vi "UHR-Fleezers Control (fpga) - avogadro 7 rm bd2.vi"() -> ()   [LabVIEW 2014]
doc: "UHR-Fleezers Instrument Control Code (fpga)"
uses:
  <vilib>/Platform/TimedLoop/XDataNode/timing_clust.ctl
  <vilib>/Platform/TimedLoop/XDataNode/nitl_modes.ctl
  <vilib>/Platform/TimedLoop/XDataNode/wakeup.ctl
  <vilib>/rvi/Emulation/niFpgaGetClockAttributes.vi
  <vilib>/rvi/Emulation/niFpgaSctlEmulationGetInTimedLoop.vi
  <vilib>/rvi/Emulation/niFpgaEmulationReportErrorSimple.vi
  <vilib>/rvi/Emulation/niFpgaProcessEmulError.vi
  <vilib>/rvi/eio/common/nirviEmuTemplateMethod_errors.vi
  <vilib>/rvi/interface/RandomDataEmulation/niFpgaRandomDataHandleErrors.vi
  <vilib>/rvi/Emulation/niFpgaCriticalErrorInLSC.vi
  <vilib>/rvi/Emulation/niFpgaEmulationIsFPGAContextNoSignature.vi
  <vilib>/rvi/errors/niFpgaSetErrorForExecOnDevCompSimple.vi
  <vilib>/rvi/eio/common/nirviEmuReportErrorAndStop.vi
  <vilib>/rvi/DataTransferAndStorage/Container/Common/niFpgaContainerGetUniqueNameForEmu.vi
  <vilib>/rvi/FIFO/Fifo_Resource/nirvififoEmulationSetSize.vi
  <vilib>/rvi/FIFO/Fifo_Resource/nirviFifoEmulationQueueMgr.vi
  <instcachedir>/0/nirviFifoEmulationQueueMgr_E5CAEC123FF24DC58D834DCA3CDAA9B5.lvgen/nirviFifoEmulationQueueMgr_E5CAEC123FF24DC58D834DCA3CDAA9B5_001.vi
  <vilib>/rvi/FIFO/Fifo_Resource/nirvififoEmulationDetermineInputValidOut.vi
  <vilib>/rvi/FIFO/Fifo_Resource/nirvififoEmulationCreateLock.vi
  <vilib>/rvi/FIFO/Fifo_Resource/nirvififoEmulationObtainLock.vi
  <vilib>/rvi/FIFO/Fifo_Resource/nirvififoEmulationReleaseLock.vi
  <vilib>/rvi/occurrence/nirviWaitOnOccurrenceBase.vi
  <vilib>/rvi/errors/nirviReportUnexpectedCaseInternalError.vi
  <vilib>/rvi/errors/nirviReportUnexpectedCaseInternalError (U32).vi
  <vilib>/rvi/DataTransferAndStorage/Container/Common/niFpgaContainerExecOnDevCompGetState.vi
  <vilib>/Utility/error.llb/Clear Errors.vi
  <vilib>/eio/EIONode/EIONode.xnode
  <vilib>/eio/EIOMethodNode/EIOMethodNode.xnode
  <vilib>/rvi/DataTransferAndStorage/Container/XNode/niFpgaContainer.xnode
  <vilib>/rvi/interface/RandomDataEmulation/nirviRandomDataFpgaReadWriteTemplate.vi
  <vilib>/rvi/FIFO/Fifo_Resource/nirvififoEmulationWrite.vi
  <vilib>/rvi/FIFO/Fifo_Resource/niFpgaFifoEmulationRefIn.vi
  <vilib>/addons/control/pid/fpga.llb/XNode/niFpgaPID.xnode
  <vilib>/Platform/TimedLoop/XDataNode/XDataNode.xnode
  <vilib>/rvi/FIFO/Fifo_Resource/nirvififoEmulationRead.vi
  <vilib>/Platform/TimedLoop/XDataNode/XDNodeRunTimeDep.lvlib
  <vilib>/rvi/Memory/Memory_Emulation/niFpgaMemoryEmulationRefIn.vi
panel:
  in  "BD 1 Delay (ticks)":u8
  out "lifetime (ticks)":u16
  in  "Lifetime to FIFO":bool
  in  "Tab Control":T1(tab)=enum."MCL trap control"
  in  "Set 3":bool
  in  "Set 2":bool=TRUE
  in  "Set 1":bool=TRUE
  in  "Trap Pos to FIFO":bool
  in  "N of AI1 Int Acq Sets":i16=2 min=1 max=3 step=1
  out "AI Late Counter":u8
  in  "ai count":u16=400
  in  "+ phase":bool
  in  "Phase count adjustment":i16
  out "Relative phase":i16
  in  "AI to FIFO":bool
  out "BD1 Frequency Out 1":u64
  out "BD1 Frequency Out 2":u64
  out "Trap Pos FIFO Timeout":u16
  out "Trap AI FIFO Timeout":u16
  in  "Trap FIFO Set Timeout":i32
  in  "Tab Control 2":T2(tab)
  in  "Multiple trap 3 position offset \nfile":bool
  in  "Piezo offset Y points":u64
  in  "Piezo offset X points":u64
  in  "Piezo offset Xmin":u64
  in  "Piezo Offset Ymin":u64
  in  "Piezo Offset Increment":u64
  out "BD1 amplitude 1 out":u16
  out "BD1 amplitude 2 out":u16
  in  "FB output range":cluster{"output low":i16, "output high":i16}={"output low"=0, "output high"=3000}
  in  "FB Gains":T3={"proportional gain (Kc)"=10, "integral gain (Kc*Ts/Ti)"=5, "derivative gain (Kc*Td/Ts)"=0}
  in  "RF synth green feedback max":i16=4000
  in  "RD":bool=TRUE
  in  "Swap F1 and F2":bool
  in  "Cont. Scan":bool
  in  "Abort scan":bool
  in  "Cycles per step":u64
  in  "Scan BD":bool
  in  "Number of scans":u16
  in  "Scan steps":u64
  in  "Scan freq.  increment":i64
  out "Scanning":bool
  in  "Start scan":bool
  in  "OSK Bd 1":bool
  in  "Reset Bd 1":bool
  in  "PMODE":bool=TRUE
  in  "Number Interlace Cycles":u8=2 min=1 max=3
  in  "Interlace Off Parameters":u8=1 min=1 max=3
  in  "Interlace ON/OFF":bool
  out "DIO Relative phase":i16
  in  "Phase count adjustment (DIO)":i16
  in  "+ phase (DIO)":bool
  out "DIO Late Counter":u8
  in  "DIO count 1 (ticks)":u16=400
  in  "DIO count 2 (ticks)":u16=400
  in  "DIO count 3 (ticks)":u16=400
  out "AI2 Y Sum Set 2":i16
  out "AI2 Y Sum Set 1":i16
  in  "FB Setpoint Set 1":i16 min=0 step=1
  in  "FB Reset Set 1":bool
  in  "FB On/Off Set 1":bool
  in  "FB Reset Set 2":bool
  in  "FB On/Off Set 2":bool
  in  "FB Setpoint Set 2":i16 min=0 step=1
  out "Scan I":u64
  in  "Amp switch delay":u8=5
  in  "RF synth bd controls green":bool
  in  "Phase Trap 2":fxp<+,14,14>
  in  "Phase Trap 1":fxp<+,14,14>
  in  "Phase offset method":u8
  in  "BD 1 Amplitude 1":u16
  in  "BD 1 Frequency 1":u64
  in  "BD 1 Amplitude 2":u16
  in  "BD 1 Frequency 2":u64
  in  "BD 1 Amplitude 3":u16
  in  "BD 1 Frequency 3":u64
  in  "Next trap write delay (ticks)":u8 caption="Count(Ticks)"
  out "Random phase generated":fxp<+,14,14>
  in  "RF phase reset before cycles":bool
  in  "Ready Write":bool
  in  "Data":i64
  in  "Address 2":u32
  out "Piezo X out":i16
  out "Piezo Y out":i16
  in  "Piezo Trap ON/Off (AO3)":i16
  in  "Piezo Trap X (AO5)":i16
  in  "Piezo Trap Y (AO4)":i16
  in  "Symmetric force feedback\nand raster scan":bool
  in  "FB Min frequency":u64
  in  "FB Max Frequency":u64
  in  "Dynamic Force FB (Ronen)":bool
  in  "Trap pos. FB Range":T4={"FB2 output low"=-1.0, "FB2 output high"=0.999969482421875}
  in  "Trap Pos. FB Gains":T5={"proportional gain (Kc)"=0.999969482421875, "integral gain (Kc*Ts/Ti)"=0.999969482421875, "derivative gain (Kc*Td/Ts)"=0.0}
  in  "B factor":fxp<+/-,32,16>
  in  "Negate Diff?":bool
  in  "Diff FB Measurement?":bool
  in  "FB Trig Integrate":u32=1
  out "TTrig?":bool
  in  "TTrig Negate Pos":bool=TRUE
  out "Trap Pos FB Int Signal":fxp<+/-,24,9> format="%.18g"
  out "Trap Pos FB Int-Norm Signal":fxp<+/-,16,1> format="%.16g"
  in  "FPGA TTrig Thresh":i64
  in  "FPGA Trap Trig":bool
  out "Trap Pos FB Action":i64
  in  "Trap Pos. FB Offset Factor":i64
  in  "Trap Pos. FB Mult Factor":i64=2
  in  "Trap Pos. FB Reset":bool
  in  "Trap Pos FB Monitor T1 or T2":bool
  in  "AI1 X Scale":u16
  in  "Trap Pos FB Int Count":u16=100
  in  "Trap Pos FB Negate Action":bool
  out "AI1 X Set 2":fxp<+/-,16,1>
  out "AI1 X Set 1":fxp<+/-,16,1>
  in  "Trap Pos. FB SP":fxp<+/-,16,1>
  in  "Force feedback":bool
  out "TTrig Sig":i64
  out "TTrig Fin Thresh":i64
  in  "ScanTrap 3 or Fl-laser":bool
  in  "1D or 2D Scan?":bool
  in  "Abort scan (MCL)":bool
  in  "MCL Scan Axis":bool
  in  "Cont. Scan (MCL)":bool
  out "Scan I (MCL)":u64
  in  "Number of scans (MCL)":u16
  out "Scanning MCL":bool
  in  "Scan steps (MCL)":u64
  in  "Cycles per step (MCL)":u64
  in  "Scan freq.  increment (MCL)":i16
  in  "Start scan (MCL)":bool
  in  "AO2 (X)":i16
  in  "AO1 (Y)":i16
  out "MCL Late Counter":u8
  in  "MCL count":u32=800
  out "MCL Relative Phase":i16
  in  "Phase count adjustment (MCL)":i16
  in  "+ phase (MCL)":bool
  in  "Lifetime events to read blue":u16=100
  in  "Lifetime read blue fifo":bool
  out "lifetime events in fifo":u16
  out "APD2 int gate":bool
  out "APD3 out state":bool
  in  "APD Gate Operating Mode":u8 max=2 step=1
  in  "Invert APD Gate":bool
  in  "APD Gate OFF Count":u16=100
  in  "APD Gate ON Count":u16=300
  out "APD 1 Gate Late Counter":u8
  out "APD 1 Gate Relative Phase":i16
  in  "Phase count adjustment (APD 1 Gate)":i16
  in  "+ phase (APD 1 Gate)":bool
  out "APD 2 Counts 0":u32
  out "APD 2 Counts 1":u32
  out "APD 1 Counts 0":u32
  out "APD 1 Counts 1":u32
  out "APD1 out state":bool
  in  "APD AO scale factor":i16=1
  in  "APD to FIFO":bool
  in  "APD Acq Rate Count":u32=20000000
  out "APD Acq Late Counter":u8
  out "APD Acq Relative Phase":i16
  in  "Phase Count Adjustment (APD Acq)":i16
  in  "+ phase (APD Acq)":bool
  in  "Phase count adjustment (APD 2 Gate)":i16
  out "APD 2 Gate Late Counter":u8
  out "APD 2 Gate Relative Phase":i16
  in  "+ phase (APD 2 Gate)":bool
  out "APD2 out state":bool
  out "APD 3 Counts 0":u32
  out "APD 3 Counts 1":u32
  out "APD 3 Gate Late Counter":u8
  in  "Phase count adjustment (APD 3 Gate)":i16
  out "APD 3 Gate Relative Phase":i16
  in  "+ phase (APD 3 Gate)":bool
  out "APD1 int gate":bool
  out "APD3 int gate":bool
  in  "Lifetime timeout APD1":u16=200
  in  "Laser choice 2":u8=100
  in  "Laser choice 1":u8=100
  in  "Laser choice 0":u8=100
  in  "FL interlace OFF count 2":u16=100
  in  "FL interlace OFF count 1":u16=100
  in  "FL interlace ON count 2":u16=300
  in  "Fl interlace ON count 1":u16=300
  in  "D3 2":i16
  in  "I3 2":i16=5
  in  "P3 2":i16=10
  in  "Green FB Setpoint 2":i16=250 min=0 step=1
  in  "Green FB Reset 2":bool
  in  "D3":i16
  in  "I3":i16=5
  in  "P3":i16=10
  in  "Green Filter Flipper":bool
  in  "Green FB Count":u16=1200
  out "Green Late Counter":u8
  out "Green FB Relative Phase":i16
  in  "Phase count adjustment (Green FB)":i16=10
  in  "+ phase (Green FB)":bool
  out "Green FB Sum":i16
  in  "Green int current ON count adj":u16=150
  in  "Current Out":u16=30000
  in  "Green FB On/Off":bool
  in  "Green FB Setpoint":i16=250 min=0 step=1
  in  "Green FB Reset":bool
  in  "Operating Mode 2":u8=2 max=2 step=1
  in  "Invert GI 2":bool
  in  "Green interlace OFF count 2":u16=900
  in  "Green interlace ON count 2":u16=300
  out "GI Late Counter 2":u8
  out "GI Relative phase 2":i16
  in  "Phase count adjustment (GI) 2":i16=20
  in  "+ phase (GI) 2":bool
  in  "FL interlace OFF count 0":u16=100
  out "GI Relative phase":i16
  in  "Phase count adjustment (GI)":i16
  in  "+ phase (GI)":bool
  in  "FL interlace ON count 0":u16=300
  out "GI Late Counter":u8
  in  "Invert GI":bool
  in  "Operating Mode":u8 max=2 step=1
  out "green FB running":bool
  in  "+ phase (RI)":bool
  out "RI Relative phase":i16
  out "RI Late Counter":u8
  in  "Red interlace ON count":u16=300
  in  "Red interlace OFF count":u16=100
  in  "Invert RI":bool
  in  "Red Laser Operating Mode":u8 max=2 step=1
  in  "Phase count adjustment (RI)":i16
  out "Red FB Intensity":i16
  in  "RI Current Out":u16=30000
  in  "Red FB On/Off":bool
  in  "D4":i16
  in  "I4":i16=5
  in  "P4":i16=10
  in  "Red FB Setpoint":i16=250 min=0 step=1
  in  "Red FB Reset":bool
  in  "RI Operating Mode 2":u8=2 max=2 step=1
  in  "Invert RI 2":bool
  in  "Phase count adjustment (BI AO)":i16=20
  in  "Blue current ON count adj (AO)":u16=150
  in  "BI Current Out":i16=30000
  in  "Blue FB On/Off":bool
  in  "D5":i16
  in  "I5":i16=5
  in  "P5":i16=10
  in  "Blue FB Setpoint":i16=250 min=0 step=1
  in  "Blue FB Reset":bool
  in  "BI Operating Mode (AO)":u8=2 max=2 step=1
  in  "Invert BI (AO)":bool
  in  "Blue OFF count (AO)":u16=900
  in  "Blue ON count (AO)":u16=300
  out "BI Late Counter (AO)":u8
  out "BI Relative phase (AO)":i16
  in  "+ phase (BI AO)":bool
  in  "Phase count adjustment (BI D)":i16
  in  "Blue Laser Operating Mode (D)":u8 max=2 step=1
  in  "Invert BI (D)":bool
  in  "Blue interlace OFF count (D)":u16=100
  in  "Blue interlace ON count (D)":u16=300
  out "Blue Late Counter (D)":u8
  out "BI Relative phase (D)":i16
  in  "+ phase (BI D)":bool
  out "Blue Intensity":i16
  in  "Invert EMCCD Gate":bool
  in  "EMCCD Gate ON count":u16=300
  in  "EMCCD Gate OFF count":u16=100
  out "EMCCD Late counter":u8
  out "EMCCD relative phase":i16
  in  "+ phase (EMCCD Gate)":bool
  in  "EMCCD Gate Operating Mode":u8 max=2 step=1
  in  "Phase Count Adjustment EMCCD Gate":i16
  # "Raster Scan AOD"
  # "1 (X)"
  # "2 (Y)"
  # "IR Intensity Feedback (RF BD 1)"
  # "FB Gains Set 1"
  # "FB output range 1"
  # "IR Intensity Feedback (RF BD 2) -\nonly when using BD 2 for green laser AOM (not trap Y)"
  # "Keep below 4096 (12 bits) to stay within range of RF board. Going over doesn't saturate, it truncates higher bits."
  # "RF phase offset control"
  # "Methods are:\n0 - Default, do nothing at all (no phase offset writes)\n1 - Manual phase adjustment\n2 - Cycle the phase adjustment using the input phase numbers as increment values for each cycle"
  # "False is usual, True is external loop method"
  # "Parameters if using the external RF switching loop"
  # "Parameters if using the usual internal RF switching method"
  # "FB Triggering Excitation Laser"
  # "Trap Pos. FB Gains"
  # "Trap Pos. FB Range"
  # "AO1 (Y)"
  # "2D"
  # "Trap 3"
  # "1D"
  # "AO2 (X)"
  # "Fl Laser"
  # "APD AO for aligning"
  # "Detection Loop"
  # "Green fluorescent laser digital gate interlacing loop"
  # "0 Forced ON\n1 Forced OFF\n2 Interlacing"
  # "ALEX settings:"
  # "Controls for usual IA ME controls green AOM"
  # "Controls for RF synth board controls green AOM"
  # "Green FB Gains"
  # "Red fluorescent laser digital gate interlacing loop"
  # "Detection Loop"
  # "0 Forced ON\n1 Forced OFF\n2 Interlacing"
  # "Analog/FB Control Loop\n(Disabled)"
  # "Digital Control Loop"
  # "Blue laser intensity reading"
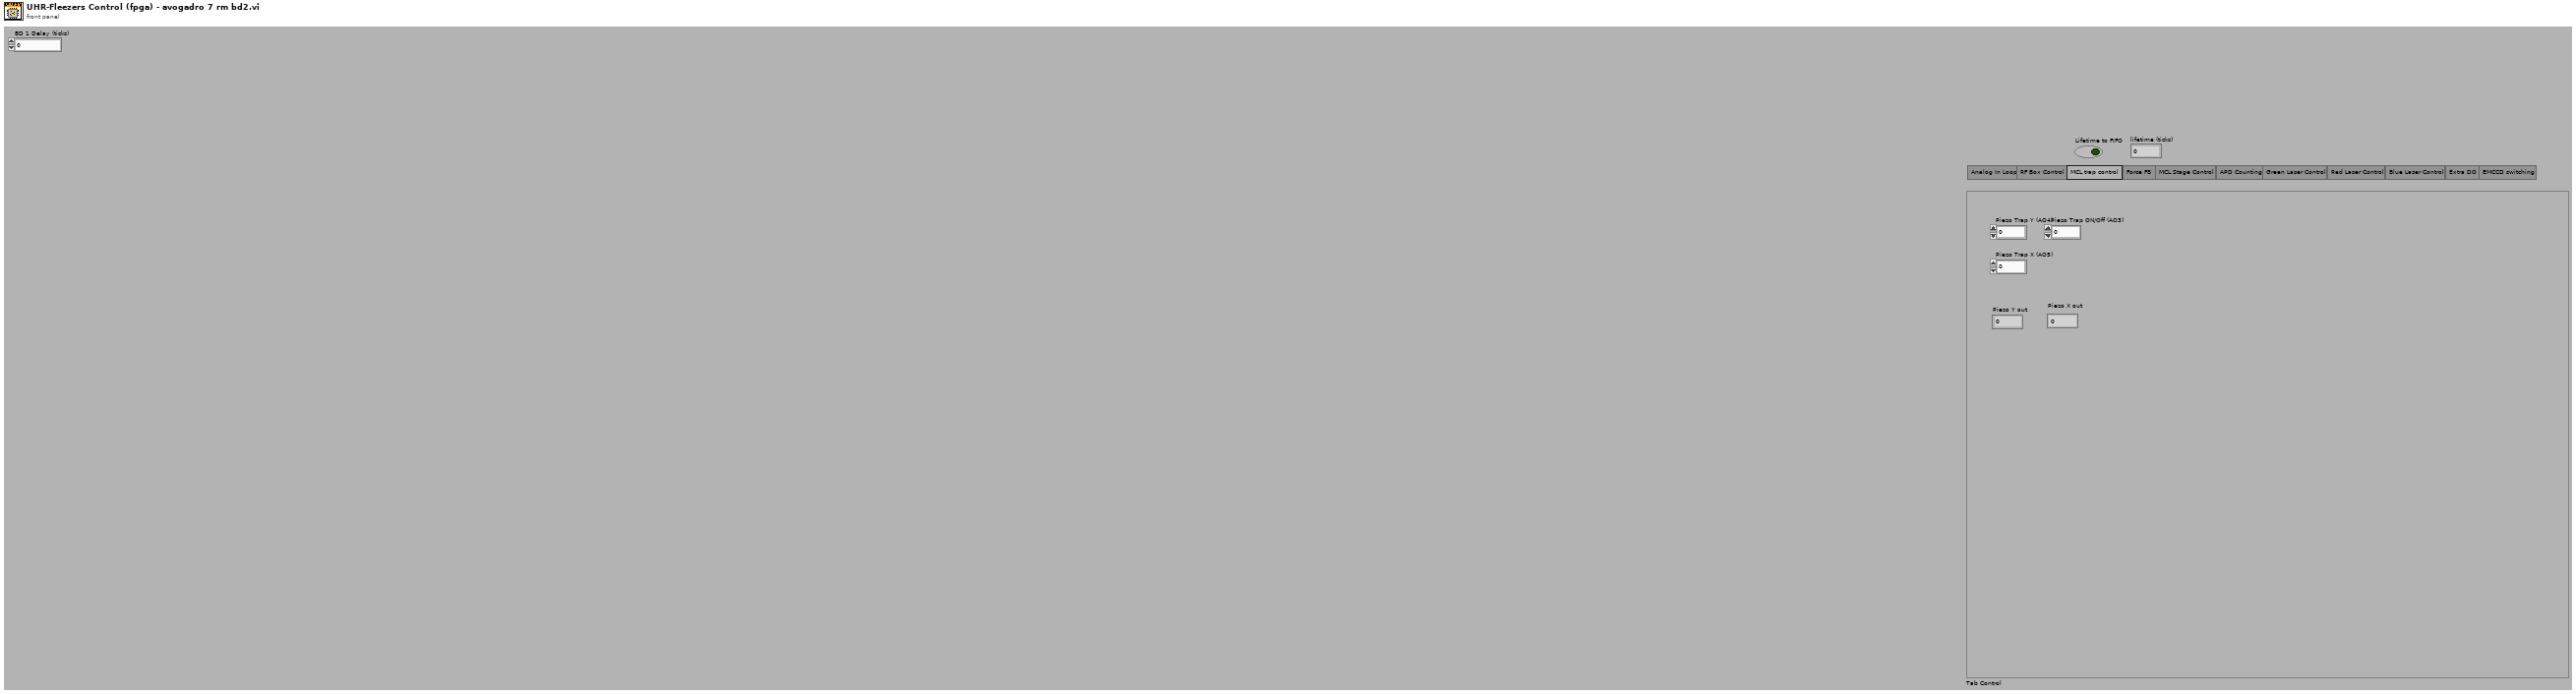
[diagram p1: front panel]
types:
  T1 = enum32{"Analog In Loop", "RF Box Control", "MCL trap control", "Force FB", "MCL Stage Control", "APD Counting", "Green Laser Control", "Red Laser Control", "Blue Laser Control", "Extra DO", "EMCCD switching"}
  T2 = enum32{"Controls", "Interlacing Frequency and Amplitude Values", "Oscillate trap from memory"}
  T3 = cluster{"proportional gain (Kc)":i16, "integral gain (Kc*Ts/Ti)":i16, "derivative gain (Kc*Td/Ts)":i16}
  T4 = cluster{"FB2 output low":fxp<+/-,16,1>, "FB2 output high":fxp<+/-,16,1>}
  T5 = cluster{"proportional gain (Kc)":fxp<+/-,16,1>, "integral gain (Kc*Ts/Ti)":fxp<+/-,16,1>, "derivative gain (Kc*Td/Ts)":fxp<+/-,16,1>}
  T6 = typedef "XDNodeRunTimeDep.lvlib/timing_clust.ctl" = cluster{"Expected End [f-1]":u64, "Actual End [f-1]":u64, "Finished Late? [f-1]":bool, "Expected End [i-1]":u64, "Actual End [i-1]":u64, "Finished Late? [i-1]":bool, "Expected Start [i]":u64, "Actual Start [i]":u64, "Expected Start [f]":u64, "Actual Start [f]":u64, "Source Name":string, "Structure Name":string, "Period":i64, "Deadline":i64, "Offset":i64, "Start":i64, "Priority":i32, "Timeout":i32, "Mode":T7, "Wakeup Reason":T8, "Error":errorcluster, "Source Type":string, "Secondary Source Type":string, "Global End Time":u64, "Global Start Time":u64, "Frame Duration":u64, "Iteration Duration":u64, "Assigned CPU":i32, "I/O Scan Engine Mode":u32}
  T7 = typedef "XDNodeRunTimeDep.lvlib/nitl_modes.ctl" = enum32{"No Change", "Process missed periods, maintain original phase", "Discard missed periods, maintain original phase", "Process missed periods, ignore original phase", "Discard missed periods, ignore original phase"}
  T8 = typedef "XDNodeRunTimeDep.lvlib/wakeup.ctl" = enum32{"Normal", "Aborted", "Asynchronous wakeup", "Timing source error", "Timed loop error", "Timeout"}
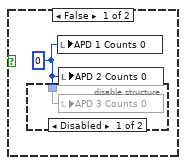
[diagram p4: hidden frame]
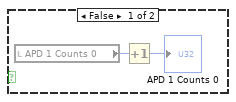
[diagram p9: hidden frame]
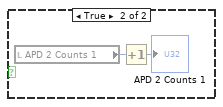
[diagram p11: hidden frame]
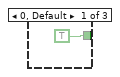
[diagram p13: hidden frame]
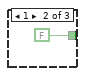
[diagram p14: hidden frame]
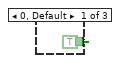
[diagram p15: hidden frame]
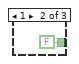
[diagram p16: hidden frame]
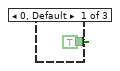
[diagram p18: hidden frame]
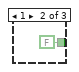
[diagram p19: hidden frame]
diagram:
  w11 = i16 0
  w15 = FALSE
  # "EMCCD gating"
  # "BD2 amp"
  # "BD1 amp"
  # "BD2 amp"
  # "BD1 amp"
  # "timing array current index"
  # "timing array"
  # "timing counter (phase adjusted here)"
  # "late counter"
  n1 = disable-structure shown="Disabled" {
    frame Disabled {
      w16 = i16 2 items=["UnSet Ready", "ReadWrite", "Wait Ready"]
      n2 = while "Handshake memory transfer for trap oscillation sin wave data" {
        shift-right: [w18] -> _
        shift-left: w16 -> [w19]
        stop <- FALSE stop-if-true
        # "Write"
        n3 = case shown="1" w19 {
          tunnel: [w22 w27 w28] -> w18
          frame 3, Default {
            w20 = i16 2 items=["UnSet Ready", "ReadWrite", "Wait Ready"]
            w21 = i16 1 items=["UnSet Ready", "ReadWrite", "Wait Ready"]
            n4 = Select(t=w21, s="Ready Write", f=w20) -> (s? t:f=w22:i16)
          }
          frame 1 {
            w27 = i16 0 items=["UnSet Ready", "ReadWrite", "Wait Ready"]
            n5 = xnode ("Memory Write")("Address"="Address 2", "Data"="Data", "Memory In"=refnum<k21> "Trap osc memory") -> ()  [unwired: 1 out]
          }
          frame 0 {
            w28 = i16 2 items=["UnSet Ready", "ReadWrite", "Wait Ready"]
            n6 = local write "Ready Write"(FALSE ("Ready Read")) -> ()
          }
        }
      }
    }
    frame Enabled {
    }
  }
  n7 = flat-sequence "FPGA initialization to do before running any of the loops" {
    tunnel: [u16 0 ("DIO count 3 (ticks)")] -> w4
    tunnel: [w34] -> _
    frame #0 {
      # "UDCLK out enable and set low"
      # "WR"
      # "BD 1"
      # "With the RF synth board initialization now done in a separate fpga vi, now when this vi is started, board is already configured and is ready for interlacing. Just need to set WR high and enabled UDCLK as write and set to low.\nbefore setting data and address bits."
      # "Start up expansion chassis early\nto avoid delays later"
      # "Set data and address values to something safe (a correct setting) so any initial WR and udclk flipping doesn't have a chance to mess anything up. Safe would be setting an unused data entry:"
      n8 = xnode "FPGA I/O Method Node"("Enable"=TRUE) -> ("FPGA I/O Out"=w31:refnum<k21>)  [unwired: 1 in]
      n9 = xnode "FPGA I/O Node"("Chassis2/Mod1/AO0"=u16 0 ("Chassis2/Mod4/AO0")) -> ("Chassis2/Mod2/AI0"=w34:i16)  [unwired: 2 in, 2 out]
      n10 = xnode "FPGA I/O Node"("Connector1/DIO15"=TRUE) -> ()  [unwired: 1 in, 1 out]
      n11 = xnode "FPGA I/O Node"("I/O Item"=FALSE ("Connector1/DIO30"), "FPGA I/O In"=w31) -> ()  [unwired: 1 out]
      n12 = xnode "FPGA I/O Node"("Connector1/DIO0"=FALSE, "Connector1/DIO1"=FALSE, "Connector1/DIO2"=FALSE, "Connector1/DIO3"=FALSE, "Connector1/DIO4"=FALSE, "Connector1/DIO5"=FALSE, "Connector1/DIO6"=FALSE, "Connector1/DIO7"=FALSE, "Connector1/DIO8"=FALSE, "Connector1/DIO9"=FALSE, "Connector1/DIO10"=FALSE, "Connector1/DIO11"=FALSE, "Connector1/DIO12"=FALSE, "Connector1/DIO13"=FALSE) -> ()  [unwired: 14 in, 14 out]
    }
  }
  n13 = node-c288() -> (w7:T6)  [unwired: 1 in]
  n14 = timed-loop "RF box board DIO control: control bits" {
    timing: w7 -> [_]
    timing-out: [_] -> w6
    tunnel: [w53] -> _
    tunnel: w4 -> [w53]
    stop <- FALSE stop-if-true
    n15 = xnode "FPGA I/O Node"("Connector1/DIO16"="RD", "Connector1/DIO17"="PMODE", "Connector1/DIO18"="OSK Bd 1", "Connector1/DIO19"="Reset Bd 1", "Connector0/DIO3"="Green Filter Flipper") -> ()  [unwired: 5 in, 5 out]
  }
  n16 = node-c288(w6) -> ()
  n17 = local read "AO1 (Y)"() -> (w13:i16)
  n18 = local read "AO2 (X)"() -> (w12:i16)
  n19 = To Unsigned Long Integer(number=w4) -> (unsigned 32bit integer=w3:u32)
  n20 = disable-structure shown="Disabled" {
    disable-tunnel: w4 -> [w61 _]
    disable-tunnel: [w60 _] -> w5
    frame Disabled {
      w60 = FALSE
      n21 = while "APD 1 Gating" {
        shift-right: [w116] -> _
        shift-left: w61 -> [w121]
        shift-right: [w115] -> _
        shift-left: w60 -> [w113]
        stop <- FALSE stop-if-true
        n22 = flat-sequence {
          tunnel: w121 -> [w124]
          tunnel: [w125] -> w119
          tunnel: [w124] -> w117
          tunnel: [w123] -> w114
          tunnel: w113 -> [w123]
          tunnel: [w128] -> w120
          tunnel: w119 -> [w128]
          tunnel: [w127] -> w118
          tunnel: w117 -> [w127]
          tunnel: w114 -> [w126]
          tunnel: [w146] -> w116
          tunnel: w120 -> [w160]
          tunnel: w118 -> [w157]
          tunnel: [w129] -> w115
          frame #0 {
            n23 = call "Loop Timer7"("Count(Ticks)"=w124) -> ("Tick Count(Ticks)"=w125:u16)
          }
          frame #1 {
            # "Signal maybe then sent through \na transistor before APD"
            n24 = xnode "FPGA I/O Node"("Connector0/DIO0"=w126) -> ()  [unwired: 1 in, 1 out]
            "APD1 int gate" <- w126
          }
          frame #2 {
            n25 = feedback #1(TRUE) -> (w152:bool)
            n26 = feedback-in #2(w160) -> ()
            n27 = feedback #2(w160) -> (w159:u16)
            n28 = Not(x=w152) -> (.not. x?=w149:bool)
            n29 = feedback-in #1(w149) -> ()
            n30 = Subtract(x=w160, y=w159) -> (x-y=w158:u16)
            n31 = Select(t="APD Gate ON Count", s=w149, f="APD Gate OFF Count") -> (s? t:f=w154:u16)
            n32 = Subtract(x=w158, y=w157) -> (x-y=w134:u16)
            n33 = Subtract(x=w154, y=w134) -> (x-y=w145:u16)
            n34 = Number To Boolean Array(number=w134) -> (Boolean array=w135:bool[])
            n35 = Or Array Elements(Boolean array=w135) -> (logical OR=w133:bool)
            n36 = Boolean To (0,1)(Boolean="+ phase (APD 1 Gate)") -> (0, 1=w143:i16)
            n37 = Boolean To (0,1)(Boolean=w133) -> (0, 1=w140:i16)
            n38 = Multiply(x=w143, y="Phase count adjustment (APD 1 Gate)") -> (x*y=w141:i16)
            n39 = To Unsigned Byte Integer(number=w140) -> (unsigned 8bit integer=w137:u8)
            n40 = Add(x=w145, y=w141) -> (x+y=w146:u16)
            n41 = feedback #3(i16 0) -> (w148:i16)
            n42 = Subtract(x=w148, y=w141) -> (x-y=w147:i16)
            "APD 1 Gate Relative Phase" <- w147
            n43 = feedback-in #3(w147) -> ()
            n44 = feedback #4(u8 0) -> (w138:u8)
            n45 = Add(x=w137, y=w138) -> (x+y=w136:u8)
            "APD 1 Gate Late Counter" <- w136
            n46 = feedback-in #4(w136) -> ()
            n47 = case shown="2" "APD Gate Operating Mode" {
              tunnel: [TRUE FALSE w163] -> w130
              tunnel: w152 -> [_ _ w163]
              frame 0, Default {
              }
              frame 1 {
              }
              frame 2 {
              }
            }
            n48 = Not(x=w130) -> (.not. x?=w131:bool)
            n49 = Select(t=w131, s="Invert APD Gate", f=w130) -> (s? t:f=w129:bool)
          }
        }
      }
      n50 = while "APD 2 Gating" {
        shift-right: [w65] -> _
        shift-left: w61 -> [w70]
        shift-right: [w64] -> _
        shift-left: w60 -> [w62]
        stop <- FALSE stop-if-true
        n51 = flat-sequence {
          tunnel: w70 -> [w73]
          tunnel: [w74] -> w68
          tunnel: [w73] -> w66
          tunnel: [w72] -> w63
          tunnel: w62 -> [w72]
          tunnel: [w77] -> w69
          tunnel: w68 -> [w77]
          tunnel: [w76] -> w67
          tunnel: w66 -> [w76]
          tunnel: w63 -> [w75]
          tunnel: [w99] -> w65
          tunnel: w69 -> [w109]
          tunnel: w67 -> [w107]
          tunnel: [w78] -> w64
          frame #0 {
            n52 = call "Loop Timer8"("Count(Ticks)"=w73) -> ("Tick Count(Ticks)"=w74:u16)
          }
          frame #1 {
            # "Signal maybe then sent through \na transistor before APD"
            n53 = xnode "FPGA I/O Node"("Connector0/DIO1"=w75) -> ()  [unwired: 1 in, 1 out]
            "APD2 int gate" <- w75
          }
          frame #2 {
            n54 = local read "APD Gate ON Count"() -> (w92:u16)
            n55 = local read "APD Gate OFF Count"() -> (w91:u16)
            n56 = feedback #5(TRUE) -> (w104:bool)
            n57 = feedback-in #6(w109) -> ()
            n58 = feedback #6(w109) -> (w93:u16)
            n59 = Not(x=w104) -> (.not. x?=w102:bool)
            n60 = feedback-in #5(w102) -> ()
            n61 = Subtract(x=w109, y=w93) -> (x-y=w108:u16)
            n62 = Select(t=w92, s=w102, f=w91) -> (s? t:f=w106:u16)
            n63 = Subtract(x=w108, y=w107) -> (x-y=w84:u16)
            n64 = Subtract(x=w106, y=w84) -> (x-y=w98:u16)
            n65 = Number To Boolean Array(number=w84) -> (Boolean array=w83:bool[])
            n66 = Or Array Elements(Boolean array=w83) -> (logical OR=w82:bool)
            n67 = Boolean To (0,1)(Boolean="+ phase (APD 2 Gate)") -> (0, 1=w96:i16)
            n68 = Multiply(x=w96, y="Phase count adjustment (APD 2 Gate)") -> (x*y=w94:i16)
            n69 = Boolean To (0,1)(Boolean=w82) -> (0, 1=w89:i16)
            n70 = Add(x=w98, y=w94) -> (x+y=w99:u16)
            n71 = To Unsigned Byte Integer(number=w89) -> (unsigned 8bit integer=w86:u8)
            n72 = feedback #7(i16 0) -> (w101:i16)
            n73 = Subtract(x=w101, y=w94) -> (x-y=w100:i16)
            "APD 2 Gate Relative Phase" <- w100
            n74 = feedback-in #7(w100) -> ()
            n75 = feedback #8(u8 0) -> (w87:u8)
            n76 = Add(x=w86, y=w87) -> (x+y=w85:u8)
            "APD 2 Gate Late Counter" <- w85
            n77 = feedback-in #8(w85) -> ()
            n78 = local read "APD Gate Operating Mode"() -> (w90:u8)
            n79 = case shown="2" w90 {
              tunnel: [TRUE FALSE w112] -> w79
              tunnel: w104 -> [_ _ w112]
              frame 0, Default {
              }
              frame 1 {
              }
              frame 2 {
              }
            }
            n80 = local read "Invert APD Gate"() -> (w81:bool)
            n81 = Not(x=w79) -> (.not. x?=w80:bool)
            n82 = Select(t=w80, s=w81, f=w79) -> (s? t:f=w78:bool)
          }
        }
      }
    }
    frame Enabled {
    }
  }
  n83 = disable-structure shown="Disabled" {
    disable-tunnel: w4 -> [w164 _]
    frame Disabled {
      n84 = while "Excitation laser intensity feedback measurement (all lasers)" {
        shift-right: [w165] -> _
        shift-left: w164 -> [w170]
        stop <- FALSE stop-if-true
        n85 = flat-sequence {
          tunnel: w170 -> [w172]
          tunnel: [w173] -> w168
          tunnel: [w172] -> w166
          tunnel: [w179] -> w169
          tunnel: w168 -> [w179]
          tunnel: [w178] -> w167
          tunnel: w166 -> [w178]
          tunnel: [w191] -> w165
          tunnel: w169 -> [w202]
          tunnel: w167 -> [w199]
          frame #0 {
            n86 = call "Loop Timer9"("Count(Ticks)"=w172) -> ("Tick Count(Ticks)"=w173:u16)
          }
          frame #1 {
            # "Design note:\n\nAll lasers need to be measured at the same \ntime because the AI expansion module\ncannot independently time the measurements\nwithin our requirements: there is dead time.\n\nThis probably wouldn't be an issue with the built\nin AI on the fpga board itself."
            n87 = xnode "FPGA I/O Node"("Connector1/DIO35"=TRUE) -> ("Chassis2/Mod1/AI2"=→"Blue Intensity", "Chassis2/Mod1/AI1"=→"Red FB Intensity", "Chassis2/Mod1/AI0"=→"Green FB Sum")  [unwired: 4 in, 4 out]
          }
          frame #2 {
            n88 = feedback-in #9(w202) -> ()
            n89 = feedback #9(w202) -> (w201:u16)
            n90 = Subtract(x=w202, y=w201) -> (x-y=w200:u16)
            n91 = xnode "FPGA I/O Node"("Connector1/DIO35"=FALSE) -> ()  [unwired: 1 in, 1 out]
            n92 = Subtract(x=w200, y=w199) -> (x-y=w181:u16)
            n93 = Subtract(x="Green FB Count", y=w181) -> (x-y=w195:u16)
            n94 = Number To Boolean Array(number=w181) -> (Boolean array=w182:bool[])
            n95 = Or Array Elements(Boolean array=w182) -> (logical OR=w180:bool)
            n96 = Boolean To (0,1)(Boolean="+ phase (Green FB)") -> (0, 1=w193:i16)
            n97 = Boolean To (0,1)(Boolean=w180) -> (0, 1=w187:i16)
            n98 = Multiply(x=w193, y="Phase count adjustment (Green FB)") -> (x*y=w188:i16)
            n99 = Add(x=w195, y=w188) -> (x+y=w191:u16)
            n100 = To Unsigned Byte Integer(number=w187) -> (unsigned 8bit integer=w184:u8)
            n101 = feedback #10(i16 0) -> (w190:i16)
            n102 = Subtract(x=w190, y=w188) -> (x-y=w189:i16)
            "Green FB Relative Phase" <- w189
            n103 = feedback-in #10(w189) -> ()
            n104 = feedback #11(u8 0) -> (w185:u8)
            n105 = Add(x=w184, y=w185) -> (x+y=w183:u8)
            "Green Late Counter" <- w183
            n106 = feedback-in #11(w183) -> ()
          }
        }
      }
    }
    frame Enabled {
    }
  }
  n107 = disable-structure shown="Disabled" {
    disable-tunnel: w4 -> [w203 _]
    frame Disabled {
      n108 = while "APD 2 Counter" {
        tunnel: w203 -> [_]
        stop <- FALSE stop-if-true
        n109 = flat-sequence {
          frame #0 {
            n110 = xnode "FPGA I/O Method Node"("FPGA I/O In"=refnum<k21> "Connector0/DIO8" ("APD 2 DO"), "Timeout"=-1) -> ()  [unwired: 2 out]
          }
          frame #1 {
            n111 = local read "APD2 int gate"() -> (w216:bool)
            n112 = case shown="True" w216 {
              frame False {
              }
              frame True {
                n113 = local read "APD2 out state"() -> (w217:bool)
                n114 = case shown="False" w217 {
                  frame False {
                    n115 = local read "APD 2 Counts 0"() -> (w219:u32)
                    n116 = Increment(x=w219) -> (x+1=→"APD 2 Counts 0":u32)
                  }
                  frame True {
                    n117 = local read "APD 2 Counts 1"() -> (w221:u32)
                    n118 = Increment(x=w221) -> (x+1=→"APD 2 Counts 1":u32)
                  }
                }
              }
            }
          }
        }
      }
      n119 = while "APD 1 Counter" {
        tunnel: w203 -> [_]
        stop <- FALSE stop-if-true
        n120 = flat-sequence {
          frame #0 {
            n121 = xnode "FPGA I/O Method Node"("FPGA I/O In"=refnum<k21> "Connector0/DIO4" ("APD 1 DO"), "Timeout"=-1) -> ()  [unwired: 2 out]
          }
          frame #1 {
            n122 = local read "APD1 int gate"() -> (w207:bool)
            n123 = case shown="True" w207 {
              frame False {
              }
              frame True {
                n124 = local read "APD1 out state"() -> (w208:bool)
                n125 = case shown="True" w208 {
                  frame False {
                    n126 = local read "APD 1 Counts 0"() -> (w210:u32)
                    n127 = Increment(x=w210) -> (x+1=→"APD 1 Counts 0":u32)
                  }
                  frame True {
                    n128 = local read "APD 1 Counts 1"() -> (w212:u32)
                    n129 = Increment(x=w212) -> (x+1=→"APD 1 Counts 1":u32)
                  }
                }
              }
            }
          }
        }
      }
    }
    frame Enabled {
    }
  }
  n130 = disable-structure shown="Disabled" {
    disable-tunnel: w4 -> [w222 _]
    frame Disabled {
      w223 = u16 0
      n131 = while "Green and red fluorescent laser interlacing (Current AO to IA 532 nm AOM ME amp)." {
        shift-right: [w303] -> _
        shift-left: w222 -> [w306]
        shift-right: [w300] -> _
        shift-left: w223 -> [w298]
        shift-right: [w297] -> _
        shift-left: w223 -> [w296]
        stop <- FALSE stop-if-true
        n132 = flat-sequence {
          tunnel: w306 -> [w310]
          tunnel: [w311] -> w305
          tunnel: [w310] -> w304
          tunnel: [w309] -> w299
          tunnel: w298 -> [w309]
          tunnel: w296 -> [w308]
          tunnel: [w308] -> w295
          tunnel: [w315] -> w302
          tunnel: w305 -> [w315]
          tunnel: [w314] -> w301
          tunnel: w304 -> [w314]
          tunnel: w299 -> [w313]
          tunnel: w295 -> [w312]
          tunnel: [w343] -> w303
          tunnel: [w359] -> w300
          tunnel: w302 -> [w370]
          tunnel: w301 -> [w367]
          tunnel: [w328] -> w297
          frame #0 {
            n133 = call "Loop Timer10"("Count(Ticks)"=w310) -> ("Tick Count(Ticks)"=w311:u16)
          }
          frame #1 {
            n134 = xnode "FPGA I/O Node"("Chassis2/Mod4/AO0"=w313, "Chassis2/Mod4/AO1"=w312) -> ()  [unwired: 2 in, 2 out]
          }
          frame #2 {
            # "IF RF synth BD does green, never run FB"
            # "ALEX variable is used by APD acquisition loop\nto turn lasers ON/OFF."
            # "Design note:\n\nThese two laser controls are in the same loop\nbecause the expansion current AI cannot separately\ntime the outputs fast enough for us.  Apparently\nit is because of communication time between the\nexpansion card and the fpga.\n\nSo the two analog control signals have the same timing\nand profile, but independent amplitudes to independently\ncontrol the intensity and feedback for each laser."
            n135 = feedback #12(TRUE) -> (w325:bool)
            n136 = Not(x=w325) -> (.not. x?=w326:bool)
            n137 = feedback-in #12(w326) -> ()
            n138 = Subtract(x="Green interlace OFF count 2", y="Green int current ON count adj") -> (x-y=w352:u16)
            n139 = feedback-in #13(w370) -> ()
            n140 = feedback #13(w370) -> (w369:u16)
            n141 = Add(x="Green int current ON count adj", y="Green interlace ON count 2") -> (x+y=w353:u16)
            n142 = Subtract(x=w370, y=w369) -> (x-y=w368:u16)
            n143 = Select(t=w353, s=w326, f=w352) -> (s? t:f=w364:u16)
            n144 = Subtract(x=w368, y=w367) -> (x-y=w336:u16)
            n145 = case shown="2" "RI Operating Mode 2" {
              tunnel: [TRUE FALSE w376] -> w321
              tunnel: w325 -> [_ _ w373]
              frame 0, Default {
              }
              frame 1 {
              }
              frame 2 {
                n146 = Not(x=w373) -> (.not. x?=w375:bool)
                n147 = Select(t=w375, s="Invert RI 2", f=w373) -> (s? t:f=w376:bool)
              }
            }
            n148 = Subtract(x=w364, y=w336) -> (x-y=w347:u16)
            n149 = case shown="2" "Operating Mode 2" {
              tunnel: [TRUE FALSE w410] -> w323
              tunnel: w325 -> [_ _ w407]
              frame 0, Default {
              }
              frame 1 {
              }
              frame 2 {
                n150 = Not(x=w407) -> (.not. x?=w409:bool)
                n151 = Select(t=w409, s="Invert GI 2", f=w407) -> (s? t:f=w410:bool)
              }
            }
            n152 = Number To Boolean Array(number=w336) -> (Boolean array=w337:bool[])
            n153 = Boolean To (0,1)(Boolean="+ phase (GI) 2") -> (0, 1=w349:i16)
            n154 = Or Array Elements(Boolean array=w337) -> (logical OR=w335:bool)
            n155 = local read item#-1() -> (w320)
            n156 = Boolean To (0,1)(Boolean=w335) -> (0, 1=w342:i16)
            n157 = Multiply(x=w349, y="Phase count adjustment (GI) 2") -> (x*y=w345:i16)
            n158 = local read item#-1() -> (w322)
            n159 = local read "RF synth bd controls green"() -> (w317:bool)
            n160 = To Unsigned Byte Integer(number=w342) -> (unsigned 8bit integer=w338:u8)
            n161 = And(x=w320, y=w321) -> (x .and. y?=w319:bool)
            n162 = Add(x=w347, y=w345) -> (x+y=w343:u16)
            n163 = feedback #14(u8 0) -> (w340:u8)
            n164 = Add(x=w338, y=w340) -> (x+y=w339:u8)
            "GI Late Counter 2" <- w339
            n165 = feedback-in #14(w339) -> ()
            n166 = feedback #15(i16 0) -> (w346:i16)
            n167 = Subtract(x=w346, y=w345) -> (x-y=w344:i16)
            "GI Relative phase 2" <- w344
            n168 = feedback-in #15(w344) -> ()
            n169 = And(x=w323, y=w322) -> (x .and. y?=w324:bool)
            n170 = And(x=w324, y="Green FB On/Off") -> (x .and. y?=w354:bool)
            "green FB running" <- w354
            n171 = And(x=w319, y="Red FB On/Off") -> (x .and. y?=w334:bool)
            n172 = Not(x=w317) -> (.not. x?=w316:bool)
            n173 = case shown="True" w334 {
              tunnel: "RI Current Out" -> [w377 _]
              tunnel: [w377 w386] -> w330
              frame False {
              }
              frame True {
                n174 = local read "Red FB Intensity"() -> (w382:i16)
                n175 = Bundle("P4"="P4", "I4"="I4", "D4"="D4") -> (w378:cluster{"P4":i16, "I4":i16, "D4":i16})  [unwired: 1 in]
                n176 = call "Slower PID.vi"("process variable"=w382, "reset?"="Red FB Reset", "setpoint"="Red FB Setpoint", "PID gains (x 2^8)"=w378, "output range"=cluster{"output high":i16, "output low":i16} {"output high"=32767, "output low"=-32768} ("Green FB output range")) -> ("output"=w389:i16)  [unwired: 10 out]
                n177 = To Long Integer(number=w389) -> (32bit integer=w383:i32)
                n178 = Add(x=w383, y=32768) -> (x+y=w385:i32)
                n179 = To Unsigned Word Integer(number=w385) -> (unsigned 16bit integer=w386:u16)
              }
            }
            n180 = And(x=w354, y=w316) -> (x .and. y?=w318:bool)
            n181 = case shown="True" w318 {
              tunnel: "Current Out" -> [w391 w392]
              tunnel: [w391 w392] -> w358
              frame False {
              }
              frame True {
                n182 = disable-structure shown="Disabled" {
                  frame Disabled {
                    n183 = local read "Green FB Sum"() -> (w397:i16)
                    n184 = Bundle("P3"="P3", "I3"="I3", "D3"="D3") -> (w393:cluster{"P3":i16, "I3":i16, "D3":i16})  [unwired: 1 in]
                    n185 = call "Slower PID.vi"("process variable"=w397, "reset?"="Green FB Reset", "setpoint"="Green FB Setpoint", "PID gains (x 2^8)"=w393, "output range"=cluster{"output high":i16, "output low":i16} {"output high"=32767, "output low"=-32768} ("Green FB output range")) -> ("output"=w403:i16)  [unwired: 10 out]
                    n186 = To Long Integer(number=w403) -> (32bit integer=w398:i32)
                    n187 = Add(x=w398, y=32768) -> (x+y=w400:i32)
                    n188 = To Unsigned Word Integer(number=w400) -> ()  [unwired: 1 out]
                  }
                  frame Enabled {
                  }
                }
              }
            }
            n189 = Boolean To (0,1)(Boolean=w319) -> (0, 1=w329:i16)
            n190 = To Unsigned Word Integer(number=w329) -> (unsigned 16bit integer=w331:u16)
            n191 = Boolean To (0,1)(Boolean=w324) -> (0, 1=w360:i16)
            n192 = To Unsigned Word Integer(number=w360) -> (unsigned 16bit integer=w357:u16)
            n193 = Compound Arithmetic op=MULTIPLY(w331, w330) -> (w328:u16)
            n194 = Compound Arithmetic op=MULTIPLY(w357, w358) -> (w359:u16)
          }
        }
      }
      n195 = while "Blue fluorescent laser interlacing (AO control direct to laser)." {
        shift-right: [w230] -> _
        shift-left: w222 -> [w233]
        shift-right: [w227] -> _
        shift-left: i16 0 -> [w225]
        stop <- FALSE stop-if-true
        n196 = flat-sequence {
          tunnel: w233 -> [w236]
          tunnel: [w237] -> w232
          tunnel: [w236] -> w231
          tunnel: [w235] -> w226
          tunnel: w225 -> [w235]
          tunnel: [w240] -> w229
          tunnel: w232 -> [w240]
          tunnel: [w239] -> w228
          tunnel: w231 -> [w239]
          tunnel: w226 -> [w238]
          tunnel: [w250] -> w230
          tunnel: [w266] -> w227
          tunnel: w229 -> [w278]
          tunnel: w228 -> [w275]
          frame #0 {
            n197 = call "Loop Timer13"("Count(Ticks)"=w236) -> ("Tick Count(Ticks)"=w237:u16)
          }
          frame #1 {
            n198 = xnode "FPGA I/O Node"("Connector0/AO3"=w238) -> ()  [unwired: 1 in, 1 out]
          }
          frame #2 {
            n199 = Subtract(x="Blue OFF count (AO)", y="Blue current ON count adj (AO)") -> (x-y=w259:u16)
            n200 = feedback-in #16(w278) -> ()
            n201 = feedback #16(w278) -> (w277:u16)
            n202 = Add(x="Blue current ON count adj (AO)", y="Blue ON count (AO)") -> (x+y=w260:u16)
            n203 = Subtract(x=w278, y=w277) -> (x-y=w276:u16)
            n204 = Subtract(x=w276, y=w275) -> (x-y=w243:u16)
            n205 = Number To Boolean Array(number=w243) -> (Boolean array=w244:bool[])
            n206 = Boolean To (0,1)(Boolean="+ phase (BI AO)") -> (0, 1=w256:i16)
            n207 = Or Array Elements(Boolean array=w244) -> (logical OR=w242:bool)
            n208 = Boolean To (0,1)(Boolean=w242) -> (0, 1=w249:i16)
            n209 = Multiply(x=w256, y="Phase count adjustment (BI AO)") -> (x*y=w252:i16)
            n210 = To Unsigned Byte Integer(number=w249) -> (unsigned 8bit integer=w245:u8)
            n211 = feedback #17(u8 0) -> (w247:u8)
            n212 = Add(x=w245, y=w247) -> (x+y=w246:u8)
            "BI Late Counter (AO)" <- w246
            n213 = feedback-in #17(w246) -> ()
            n214 = feedback #18(i16 0) -> (w253:i16)
            n215 = Subtract(x=w253, y=w252) -> (x-y=w251:i16)
            "BI Relative phase (AO)" <- w251
            n216 = feedback-in #18(w251) -> ()
            n217 = feedback #19(TRUE) -> (w270:bool)
            n218 = case shown="2" "BI Operating Mode (AO)" {
              tunnel: [TRUE FALSE w294] -> w261
              tunnel: w270 -> [_ _ w291]
              frame 0, Default {
              }
              frame 1 {
              }
              frame 2 {
                n219 = Not(x=w291) -> (.not. x?=w293:bool)
                n220 = Select(t=w293, s="Invert BI (AO)", f=w291) -> (s? t:f=w294:bool)
              }
            }
            n221 = And(x=w261, y="Blue FB On/Off") -> (x .and. y?=w262:bool)
            n222 = case shown="True" w262 {
              tunnel: "BI Current Out" -> [w279 _]
              tunnel: [w279 w281] -> w265
              frame False {
              }
              frame True {
                n223 = local read "Blue Intensity"() -> (w280:i16)
                n224 = Bundle("P5"="P5", "I5"="I5", "D5"="D5") -> (w282:cluster{"P5":i16, "I5":i16, "D5":i16})  [unwired: 1 in]
                n225 = call "Slower PID.vi"("process variable"=w280, "reset?"="Blue FB Reset", "setpoint"="Blue FB Setpoint", "PID gains (x 2^8)"=w282, "output range"=cluster{"output high":i16, "output low":i16} {"output high"=32767, "output low"=0} ("Green FB output range")) -> ("output"=w281:i16)  [unwired: 10 out]
              }
            }
            n226 = Not(x=w270) -> (.not. x?=w267:bool)
            n227 = Select(t=w260, s=w267, f=w259) -> (s? t:f=w272:u16)
            n228 = Subtract(x=w272, y=w243) -> (x-y=w254:u16)
            n229 = Add(x=w254, y=w252) -> (x+y=w250:u16)
            n230 = feedback-in #19(w267) -> ()
            n231 = Boolean To (0,1)(Boolean=w261) -> (0, 1=w241:i16)
            n232 = Multiply(x=w241, y=w265) -> (x*y=w266:i16)
          }
        }
      }
    }
    frame Enabled {
    }
  }
  n233 = while "fluorescent laser interlacing (DO)." {
    shift-right: [w417] -> _
    shift-left: w4 -> [w422]
    shift-right: [w416] -> _
    shift-left: w15 -> [w414]
    shift-right: [w413] -> _
    shift-left: u8 0 -> [w411]
    stop <- FALSE stop-if-true
    n234 = flat-sequence {
      tunnel: w422 -> [w426]
      tunnel: [w427] -> w420
      tunnel: [w426] -> w418
      tunnel: [w425] -> w415
      tunnel: w414 -> [w425]
      tunnel: [w424] -> w412
      tunnel: w411 -> [w424]
      tunnel: [w431] -> w421
      tunnel: w420 -> [w431]
      tunnel: [w430] -> w419
      tunnel: w418 -> [w430]
      tunnel: w415 -> [w429]
      tunnel: w412 -> [w428]
      tunnel: [w460] -> w417
      tunnel: w421 -> [w479]
      tunnel: w419 -> [w476]
      tunnel: [w469] -> w416
      tunnel: [w442] -> w413
      frame #0 {
        n235 = call "Loop Timer4"("Count(Ticks)"=w426) -> ("Tick Count(Ticks)"=w427:u16)
      }
      frame #1 {
        n236 = case shown="0, Default" w428 {
          tunnel: w429 -> [w433 w435 w437]
          frame 0, Default {
            w432 = FALSE
            n237 = xnode "FPGA I/O Node"("Connector0/DIO9"=w433, "Connector0/DIO11"=w432, "Connector0/DIO13"=w432) -> ()  [unwired: 3 in, 3 out]
          }
          frame 1 {
            w434 = FALSE
            n238 = xnode "FPGA I/O Node"("Connector0/DIO9"=w434, "Connector0/DIO11"=w435, "Connector0/DIO13"=w434) -> ()  [unwired: 3 in, 3 out]
          }
          frame 2 {
            w436 = FALSE
            n239 = xnode "FPGA I/O Node"("Connector0/DIO9"=w436, "Connector0/DIO11"=w436, "Connector0/DIO13"=w437) -> ()  [unwired: 3 in, 3 out]
          }
        }
      }
      frame #2 {
        # "Laser counting"
        n240 = feedback-in #20(w479) -> ()
        n241 = feedback #20(w479) -> (w478:u16)
        n242 = Subtract(x=w479, y=w478) -> (x-y=w477:u16)
        n243 = Subtract(x=w477, y=w476) -> (x-y=w438:u16)
        n244 = Number To Boolean Array(number=w438) -> (Boolean array=w454:bool[])
        n245 = Or Array Elements(Boolean array=w454) -> (logical OR=w453:bool)
        n246 = Equal To 0?(x=w438) -> ()  [unwired: 1 out]
        n247 = feedback #21(u8 0) -> (w451:u8)
        n248 = Increment(x=w451) -> (x+1=w448:u8)
        n249 = Less?(x=u8 5, y=w448) -> (x < y?=w449:bool)
        n250 = Select(t=u8 0, s=w449, f=w448) -> (s? t:f=w440:u8)
        n251 = feedback-in #21(w440) -> ()
        n252 = Boolean To (0,1)(Boolean=w453) -> (0, 1=w459:i16)
        n253 = Quotient & Remainder(x=w440, y=u8 2) -> (floor(x/y)=w439:u8)  [unwired: 1 out]
        n254 = To Unsigned Byte Integer(number=w459) -> (unsigned 8bit integer=w456:u8)
        n255 = feedback #22(u8 0) -> (w457:u8)
        n256 = Add(x=w456, y=w457) -> (x+y=w455:u8)
        "GI Late Counter" <- w455
        n257 = feedback-in #22(w455) -> ()
        n258 = Boolean To (0,1)(Boolean="+ phase (GI)") -> (0, 1=w465:i16)
        n259 = Multiply(x=w465, y="Phase count adjustment (GI)") -> (x*y=w462:i16)
        n260 = feedback #23(i16 0) -> (w463:i16)
        n261 = Subtract(x=w463, y=w462) -> (x-y=w461:i16)
        "GI Relative phase" <- w461
        n262 = feedback-in #23(w461) -> ()
        n263 = feedback #24(TRUE) -> (w472:bool)
        n264 = case shown="2" "Operating Mode" {
          tunnel: [TRUE FALSE w569] -> w469
          tunnel: w472 -> [_ _ w566]
          frame 0, Default {
          }
          frame 1 {
          }
          frame 2 {
            n265 = Not(x=w566) -> (.not. x?=w568:bool)
            n266 = Select(t=w568, s="Invert GI", f=w566) -> (s? t:f=w569:bool)
          }
        }
        n267 = Not(x=w472) -> (.not. x?=w468:bool)
        n268 = case shown="0, Default" w439 {
          tunnel: "FL interlace ON count 0" -> [w489 w516 w543]
          tunnel: "FL interlace OFF count 0" -> [w488 w515 w542]
          tunnel: w468 -> [w487 w514 w545]
          tunnel: [w485 w513 w541] -> w466
          tunnel: w438 -> [w486 w517 w544]
          tunnel: "Fl interlace ON count 1" -> [w484 w512 w540]
          tunnel: "FL interlace OFF count 1" -> [w483 w511 w539]
          tunnel: "FL interlace ON count 2" -> [w482 w510 w538]
          tunnel: "FL interlace OFF count 2" -> [w481 w509 w537]
          tunnel: ["Laser choice 0" "Laser choice 1" "Laser choice 2"] -> w442
          frame 0, Default {
            n269 = case shown="1" "Laser choice 0" {
              tunnel: w489 -> [w494 _ _]
              tunnel: w488 -> [w493 _ _]
              tunnel: w487 -> [w492 w498 w504]
              tunnel: w486 -> [w491 w497 w503]
              tunnel: [w490 w496 w502] -> w485
              tunnel: w484 -> [_ w500 _]
              tunnel: w483 -> [_ w499 _]
              tunnel: w482 -> [_ _ w506]
              tunnel: w481 -> [_ _ w505]
              frame 0, Default {
                n270 = Select(t=w494, s=w492, f=w493) -> (s? t:f=w495:u16)
                n271 = Subtract(x=w495, y=w491) -> (x-y=w490:u16)
              }
              frame 1 {
                n272 = Select(t=w500, s=w498, f=w499) -> (s? t:f=w501:u16)
                n273 = Subtract(x=w501, y=w497) -> (x-y=w496:u16)
              }
              frame 2 {
                n274 = Select(t=w506, s=w504, f=w505) -> (s? t:f=w507:u16)
                n275 = Subtract(x=w507, y=w503) -> (x-y=w502:u16)
              }
            }
          }
          frame 1 {
            n276 = case shown="0, Default" "Laser choice 1" {
              tunnel: w516 -> [w522 _ _]
              tunnel: w515 -> [w521 _ _]
              tunnel: w514 -> [w520 w526 w532]
              tunnel: w517 -> [w519 w525 w531]
              tunnel: [w518 w524 w530] -> w513
              tunnel: w512 -> [_ w528 _]
              tunnel: w511 -> [_ w527 _]
              tunnel: w510 -> [_ _ w534]
              tunnel: w509 -> [_ _ w533]
              frame 0, Default {
                n277 = Select(t=w522, s=w520, f=w521) -> (s? t:f=w523:u16)
                n278 = Subtract(x=w523, y=w519) -> (x-y=w518:u16)
              }
              frame 1 {
                n279 = Select(t=w528, s=w526, f=w527) -> (s? t:f=w529:u16)
                n280 = Subtract(x=w529, y=w525) -> (x-y=w524:u16)
              }
              frame 2 {
                n281 = Select(t=w534, s=w532, f=w533) -> (s? t:f=w535:u16)
                n282 = Subtract(x=w535, y=w531) -> (x-y=w530:u16)
              }
            }
          }
          frame 2 {
            n283 = case shown="1" "Laser choice 2" {
              tunnel: w543 -> [w550 _ _]
              tunnel: w542 -> [w549 _ _]
              tunnel: w545 -> [w548 w554 w560]
              tunnel: w544 -> [w547 w553 w559]
              tunnel: [w546 w552 w558] -> w541
              tunnel: w540 -> [_ w556 _]
              tunnel: w539 -> [_ w555 _]
              tunnel: w538 -> [_ _ w562]
              tunnel: w537 -> [_ _ w561]
              frame 0, Default {
                n284 = Select(t=w550, s=w548, f=w549) -> (s? t:f=w551:u16)
                n285 = Subtract(x=w551, y=w547) -> (x-y=w546:u16)
              }
              frame 1 {
                n286 = Select(t=w556, s=w554, f=w555) -> (s? t:f=w557:u16)
                n287 = Subtract(x=w557, y=w553) -> (x-y=w552:u16)
              }
              frame 2 {
                n288 = Select(t=w562, s=w560, f=w561) -> (s? t:f=w563:u16)
                n289 = Subtract(x=w563, y=w559) -> (x-y=w558:u16)
              }
            }
          }
        }
        n290 = Add(x=w466, y=w462) -> (x+y=w460:u16)
        n291 = feedback-in #24(w468) -> ()
      }
    }
  }
  n292 = while "DAQ AI set 1" {
    shift-right: [w570] -> _
    shift-left: w4 -> [w575]
    stop <- FALSE stop-if-true
    n293 = flat-sequence {
      tunnel: w575 -> [w585]
      tunnel: [w586] -> w573
      tunnel: [w585] -> w572
      tunnel: [w596] -> w583
      tunnel: [w595] -> w582
      tunnel: [w594] -> w581
      tunnel: [w593] -> w580
      tunnel: [w592] -> w579
      tunnel: [w591] -> w578
      tunnel: [w590] -> w577
      tunnel: [w589] -> w576
      tunnel: [w588] -> w574
      tunnel: w573 -> [w588]
      tunnel: w572 -> [w587]
      tunnel: [w587] -> w571
      tunnel: [w628] -> w570
      tunnel: w583 -> [w654]
      tunnel: w582 -> [w620]
      tunnel: w581 -> [w621]
      tunnel: w580 -> [w598]
      tunnel: w579 -> [w644]
      tunnel: w578 -> [w643]
      tunnel: w577 -> [w642]
      tunnel: w576 -> [w641]
      tunnel: w574 -> [w638]
      tunnel: w571 -> [w635]
      frame #0 {
        n294 = call "Loop Timer3"("Count(Ticks)"=w585) -> ("Tick Count(Ticks)"=w586:u16)
      }
      frame #1 {
        # "Signal changed to DIO15 to ease\nmeasurement in the room - change\nback for large code"
        n295 = xnode "FPGA I/O Node"("Connector0/DIO15"=TRUE ("Connector1/DIO33")) -> ("Connector0/AI0"=w596:i16, "Connector0/AI1"=w595:i16, "Connector0/AI2"=w594:i16, "Connector0/AI3"=w593:i16, "Connector0/AI4"=w592:i16, "Connector0/AI5"=w591:i16, "Connector0/AI6"=w590:i16, "Connector0/AI7"=w589:i16)  [unwired: 9 in, 9 out]
      }
      frame #2 {
        w624 = FALSE ("AI to FIFO")
        # "Normalize by trap bead QPD sum, AI3"
        # "Adjust phase after data acquired if button pressed"
        n296 = feedback #25(i16 1) -> (w647:i16)
        n297 = Increment(x=w647) -> (x+1=w653:i16)
        n298 = Scale By Power Of 2(n="AI1 X Scale", x=w620) -> (x*2^n=w618:i16)
        n299 = Greater?(x=w653, y="N of AI1 Int Acq Sets") -> (0:w650:bool)
        n300 = Select(t=i16 1, s=w650, f=w653) -> (s? t:f=w652:i16)
        n301 = feedback-in #25(w652) -> ()
        n302 = Divide(x=w618, y=w598) -> (x/y=w617:fxp<+/-,16,1>)
        n303 = feedback #26(w624) -> (w622:bool)
        n304 = feedback #27(w624) -> (w640:bool)
        n305 = case shown="1, Default" w647 {
          tunnel: w621 -> [w679 w686 _]
          tunnel: ["Set 1" "Set 2" "Set 3"] -> w645
          tunnel: ["AI to FIFO" w688 w693] -> w639
          tunnel: w640 -> [_ w688 w693]
          tunnel: ["Trap Pos to FIFO" w687 w692] -> w623
          tunnel: w622 -> [_ w687 w692]
          tunnel: w617 -> [w678 w685 _]
          tunnel: [w677 w683 FALSE] -> w604
          tunnel: [w676 w684 u64 0 ("BD1 Frequency Out 2")] -> w603
          frame 1, Default {
            n306 = local read "BD1 Frequency Out 1"() -> (w676:u64)
            n307 = Compound Arithmetic op=AND("Trap Pos to FIFO", "Set 1", "AI to FIFO") -> (w677:bool)
            "AI2 Y Sum Set 1" <- w679
            "AI1 X Set 1" <- w678
          }
          frame 2 {
            n308 = local read "BD1 Frequency Out 2"() -> (w684:u64)
            n309 = Compound Arithmetic op=AND(w687, "Set 2", w688) -> (w683:bool)
            "AI2 Y Sum Set 2" <- w686
            "AI1 X Set 2" <- w685
          }
          frame 3 {
          }
        }
        n310 = And(x=w645, y=w639) -> (x .and. y?=w646:bool)
        n311 = case shown="True" w646 {
          tunnel: w654 -> [_ w707]
          tunnel: w620 -> [_ w706]
          tunnel: w621 -> [_ w705]
          tunnel: w598 -> [_ w704]
          tunnel: w644 -> [_ w703]
          tunnel: w643 -> [_ w702]
          tunnel: w642 -> [_ w701]
          tunnel: w641 -> [_ w700]
          tunnel: 0 ("DMA buffer timeout") -> [_ w709]
          frame False {
          }
          frame True {
            n312 = Build Array(w707, w706, w705, w704, w703, w702, w701, w700) -> (w708:i16[])
            n313 = for {
              tunnel: w708 -> [w711] mode=indexing
              tunnel: w709 -> [w712]
              tunnel: [w710] -> w698 mode=indexing
              n314 = xnode ("FIFO Write")("Element"=w711, "Timeout"=w712) -> ("Timed Out?"=w710:bool)  [unwired: 1 in, 1 out]
            }
            n315 = Or Array Elements(Boolean array=w698) -> (logical OR=w695:bool)
            n316 = Boolean To (0,1)(Boolean=w695) -> (0, 1=w697:i16)
            n317 = feedback #28(u16 0) -> (w696:u16)
            n318 = Add(x=w697, y=w696) -> (x+y=w694:u16)
            "Trap AI FIFO Timeout" <- w694
            n319 = feedback-in #28(w694) -> ()
          }
        }
        n320 = feedback-in #26(w623) -> ()
        n321 = feedback-in #27(w639) -> ()
        n322 = local read "Piezo X out"() -> (w600:i16)
        n323 = local read "Piezo Y out"() -> (w599:i16)
        n324 = case shown="True" w604 {
          tunnel: w603 -> [_ w662]
          tunnel: [u8 0 w659] -> w602
          tunnel: w600 -> [_ w658]
          tunnel: w599 -> [_ w657]
          frame False {
          }
          frame True {
            n325 = Split Number(x=w662) -> (hi(x)=w663:u32, lo(x)=w664:u32)
            n326 = Split Number(x=w663) -> (lo(x)=w665:u16)  [unwired: 1 out]
            n327 = Split Number(x=w664) -> (hi(x)=w666:u16, lo(x)=w667:u16)
            n328 = Build Array "BD 1 nu Stack"(w665, w666, w667, w658, w657) -> (w661:u16[])
            n329 = for {
              tunnel: w661 -> [w674] mode=indexing
              shift-right: [w670] -> w659
              shift-left: u8 0 -> [w671]
              n330 = xnode ("FIFO Method Node")("Element"=w674, "Timeout"="Trap FIFO Set Timeout") -> ("Timed Out?"=w673:bool)  [unwired: 1 in, 1 out]
              n331 = Boolean To (0,1)(Boolean=w673) -> (0, 1=w672:i16)
              n332 = To Unsigned Byte Integer(number=w672) -> (unsigned 8bit integer=w669:u8)
              n333 = Add(x=w669, y=w671) -> (x+y=w670:u8)
            }
          }
        }
        n334 = To Unsigned Word Integer(number=w602) -> (unsigned 16bit integer=w601:u16)
        n335 = feedback #29(u16 0) -> (w615:u16)
        n336 = Add(x=w601, y=w615) -> (x+y=w614:u16)
        "Trap Pos FIFO Timeout" <- w614
        n337 = feedback-in #29(w614) -> ()
        n338 = feedback-in #30(w638) -> ()
        n339 = feedback #30(w638) -> (w637:u16)
        n340 = Subtract(x=w638, y=w637) -> (x-y=w636:u16)
        n341 = xnode "FPGA I/O Node"("Connector0/DIO15"=FALSE ("Connector1/DIO34")) -> ()  [unwired: 1 in, 1 out]
        n342 = Subtract(x=w636, y=w635) -> (x-y=w606:u16)
        n343 = Boolean To (0,1)(Boolean="+ phase") -> (0, 1=w631:i16)
        n344 = Multiply(x=w631, y="Phase count adjustment") -> (x*y=w625:i16)
        n345 = Subtract(x="ai count", y=w606) -> (x-y=w629:u16)
        n346 = Number To Boolean Array(number=w606) -> (Boolean array=w607:bool[])
        n347 = feedback #31(i16 0) -> (w627:i16)
        n348 = Add(x=w629, y=w625) -> (x+y=w628:u16)
        n349 = Subtract(x=w627, y=w625) -> (x-y=w626:i16)
        "Relative phase" <- w626
        n350 = feedback-in #31(w626) -> ()
        n351 = Or Array Elements(Boolean array=w607) -> (logical OR=w605:bool)
        n352 = Boolean To (0,1)(Boolean=w605) -> (0, 1=w612:i16)
        n353 = To Unsigned Byte Integer(number=w612) -> (unsigned 8bit integer=w609:u8)
        n354 = feedback #32(u8 0) -> (w610:u8)
        n355 = Add(x=w609, y=w610) -> (x+y=w608:u8)
        "AI Late Counter" <- w608
        n356 = feedback-in #32(w608) -> ()
      }
    }
  }
  n357 = while "MCL stage control" {
    shift-right: [w736] -> _
    shift-left: w4 -> [w739]
    shift-right: [w729] -> _
    shift-left: w13 -> [w726]
    shift-right: [w728] -> _
    shift-left: w12 -> [w724]
    shift-right: [w723] -> _
    shift-left: w11 -> [w718]
    shift-right: [w721] -> _
    shift-left: w11 -> [w713]
    shift-right: [w719] -> _
    shift-left: w11 -> [w715]
    stop <- FALSE stop-if-true
    n358 = flat-sequence {
      tunnel: w739 -> [w746]
      tunnel: [w747] -> w735
      tunnel: [w746] -> w733
      tunnel: [w745] -> w727
      tunnel: w726 -> [w745]
      tunnel: [w744] -> w725
      tunnel: w724 -> [w744]
      tunnel: w718 -> [w743]
      tunnel: [w743] -> w717
      tunnel: [w742] -> w716
      tunnel: w715 -> [w742]
      tunnel: [w741] -> w714
      tunnel: w713 -> [w741]
      tunnel: w735 -> [w754]
      tunnel: [w754] -> w734
      tunnel: w733 -> [w753]
      tunnel: [w753] -> w732
      tunnel: w727 -> [w752]
      tunnel: w725 -> [w751]
      tunnel: w717 -> [w750]
      tunnel: w716 -> [w749]
      tunnel: w714 -> [w748]
      tunnel: w734 -> [w768]
      tunnel: w732 -> [w767]
      tunnel: [w768] -> w738
      tunnel: [w767] -> w737
      tunnel: [w766] -> w731
      tunnel: [w765] -> w730
      tunnel: [w757] -> w722
      tunnel: [w755] -> w720
      tunnel: [w875] -> w736
      tunnel: w738 -> [w882]
      tunnel: w737 -> [w879]
      tunnel: w731 -> [w877]
      tunnel: w730 -> [w876]
      tunnel: [w877] -> w729
      tunnel: [w876] -> w728
      tunnel: [w858] -> w723
      tunnel: w722 -> [w858]
      tunnel: [w857] -> w721
      tunnel: w720 -> [w857]
      tunnel: ["Piezo Trap ON/Off (AO3)"] -> w719
      frame #0 {
        n359 = call "Loop Timer5"("Count(Ticks)"=w746) -> ("Tick Count(Ticks)"=w747:u32)
      }
      frame #1 {
        n360 = xnode "FPGA I/O Node"("Connector0/AO1"=w752, "Connector0/AO2"=w751, "Connector0/AO3"=w749, "Connector0/AO4"=w750, "Connector0/AO5"=w748) -> ()  [unwired: 5 in, 5 out]
      }
      frame #2 {
        n361 = local read "Scanning MCL"() -> (w780:bool)
        n362 = Or(x=w780, y="Start scan (MCL)") -> (x .or. y?=w775:bool)
        n363 = Not(x="Abort scan (MCL)") -> (.not. x?=w773:bool)
        n364 = And(x=w773, y=w775) -> (x .and. y?=w772:bool)
        n365 = case "Raster scan" shown="False" w772 {
          tunnel: [w813 w856] -> w777
          tunnel: "Start scan (MCL)" -> [_ w841]
          tunnel: [w813 w817] -> w761
          frame False {
            w813 = i16 0
            n366 = local write "Scanning MCL"(FALSE ("scanning")) -> ()
          }
          frame True {
            w827 = i16 0
            w826 = u64 0
            # "scan incr."
            # "freq. incr. mult."
            # "count steps"
            # "count number of cycles"
            n367 = feedback #33(w826) -> (w853:u64)
            n368 = Select(t=w826, s=w841, f=w853) -> (s? t:f=w855:u64)
            n369 = Increment(x=w855) -> (x+1=w852:u64)
            n370 = Greater?(x="Cycles per step (MCL)", y=w852) -> (0:w836:bool)
            n371 = Select(t=w852, s=w836, f=w826) -> (s? t:f=w851:u64)
            n372 = feedback-in #33(w851) -> ()
            n373 = feedback #34(w826) -> (w850:u64)
            n374 = Select(t=w826, s=w841, f=w850) -> (s? t:f=w845:u64)
            n375 = Increment(x=w845) -> (x+1=w849:u64)
            n376 = Add(x="Scan steps (MCL)", y="Scan steps (MCL)") -> (x+y=w848:u64)
            n377 = Select(t=w845, s=w836, f=w849) -> (s? t:f=w831:u64)
            n378 = Greater?(x=w848, y=w831) -> (0:w830:bool)
            n379 = Select(t=w831, s=w830, f=w826) -> (s? t:f=w846:u64)
            n380 = feedback-in #34(w846) -> ()
            n381 = Equal?(x="Scan steps (MCL)", y=w831) -> (x = y?=w835:bool)
            n382 = Greater?(x="Scan steps (MCL)", y=w845) -> (0:w844:bool)
            n383 = feedback #35(w827) -> (w847:i16)
            n384 = Select(t=w827, s=w841, f=w847) -> (s? t:f=w833:i16)
            n385 = Increment(x=w833) -> (x+1=w843:i16)
            n386 = Decrement(x=w833) -> (x-1=w842:i16)
            n387 = Select(t=w843, s=w844, f=w842) -> (s? t:f=w834:i16)
            n388 = Select(t=w833, s=w835, f=w834) -> (s? t:f=w832:i16)
            n389 = Select(t=w833, s=w836, f=w832) -> (s? t:f=w828:i16)
            n390 = Select(t=w828, s=w830, f=w827) -> (s? t:f=w829:i16)
            n391 = feedback-in #35(w829) -> ()
            n392 = feedback #36(w826) -> (w840:u64)
            n393 = Select(t=w826, s=w841, f=w840) -> (s? t:f=w815:u64)
            n394 = Increment(x=w815) -> (x+1=w837:u64)
            n395 = Select(t=w815, s=w830, f=w837) -> (s? t:f=w816:u64)
            n396 = Greater?(x="Number of scans (MCL)", y=w816) -> (0:w823:bool)
            n397 = Multiply(x="Scan freq.  increment (MCL)", y=w833) -> (x*y=w856:i16)
            n398 = Select(t=TRUE, s="Cont. Scan (MCL)", f=w823) -> (s? t:f=w822:bool)
            "Scanning MCL" <- w822
            n399 = Select(t=w816, s=w822, f=w826) -> (s? t:f=w838:u64)
            n400 = feedback-in #36(w838) -> ()
            n401 = Increment(x=w816) -> (x+1=→"Scan I (MCL)":u64)
            n402 = To Word Integer(number=w815) -> (16bit integer=w818:i16)
            n403 = Multiply(x=w818, y="Scan freq.  increment (MCL)") -> (x*y=w817:i16)
          }
        }
        n404 = case shown="True" "Multiple trap 3 position offset \nfile" {
          tunnel: ["Piezo Trap Y (AO4)" w800] -> w758
          tunnel: ["Piezo Trap X (AO5)" w799] -> w756
          frame False {
          }
          frame True {
            n405 = local read "Scan I"() -> (w811:u64)
            n406 = Decrement(x=w811) -> (x-1=w812:u64)
            n407 = Quotient & Remainder(x=w812, y="Piezo offset Y points") -> (x-y*floor(x/y)=w809:u64, floor(x/y)=w807:u64)
            n408 = Multiply(x=w809, y="Piezo Offset Increment") -> (x*y=w806:u64)
            n409 = Multiply(x="Piezo Offset Increment", y=w807) -> (x*y=w804:u64)
            n410 = Add(x=w804, y="Piezo offset Xmin") -> (x+y=w801:u64)
            n411 = Add(x=w806, y="Piezo Offset Ymin") -> (x+y=w802:u64)
            n412 = To Word Integer(number=w801) -> (16bit integer=w799:i16)
            n413 = To Word Integer(number=w802) -> (16bit integer=w800:i16)
          }
        }
        n414 = Select(t=w761, s="1D or 2D Scan?", f=i16 0) -> (s? t:f=w762:i16)
        n415 = Select(t=w777, s="MCL Scan Axis", f=w762) -> (s? t:f=w778:i16)
        n416 = Select(t=w762, s="MCL Scan Axis", f=w777) -> (s? t:f=w776:i16)
        n417 = case shown="True" "ScanTrap 3 or Fl-laser" {
          tunnel: w778 -> [w788 w790]
          tunnel: w776 -> [w783 w794]
          tunnel: "AO2 (X)" -> [w784 w795]
          tunnel: "AO1 (Y)" -> [w787 w796]
          tunnel: [w786 w796] -> w766
          tunnel: [w785 w795] -> w765
          tunnel: w758 -> [w782 w791]
          tunnel: [w782 w789] -> w757
          tunnel: w756 -> [w781 w793]
          tunnel: [w781 w792] -> w755
          frame False {
            n418 = Add(x=w784, y=w783) -> (x+y=w785:i16)
            n419 = Add(x=w787, y=w788) -> (x+y=w786:i16)
          }
          frame True {
            n420 = Add(x=w791, y=w790) -> (x+y=w789:i16)
            n421 = Add(x=w793, y=w794) -> (x+y=w792:i16)
          }
        }
      }
      frame #3 {
        n422 = feedback-in #37(w882) -> ()
        n423 = feedback #37(w882) -> (w881:u32)
        n424 = Boolean To (0,1)(Boolean="+ phase (MCL)") -> (0, 1=w873:i16)
        n425 = Subtract(x=w882, y=w881) -> (x-y=w880:u32)
        n426 = Multiply(x=w873, y="Phase count adjustment (MCL)") -> (x*y=w869:i16)
        n427 = Subtract(x=w880, y=w879) -> (x-y=w861:u32)
        n428 = Subtract(x="MCL count", y=w861) -> (x-y=w871:u32)
        n429 = feedback #38(i16 0) -> (w870:i16)
        n430 = Subtract(x=w870, y=w869) -> (x-y=w868:i16)
        "MCL Relative Phase" <- w868
        n431 = feedback-in #38(w868) -> ()
        n432 = Number To Boolean Array(number=w861) -> (Boolean array=w862:bool[])
        n433 = Or Array Elements(Boolean array=w862) -> (logical OR=w860:bool)
        n434 = Boolean To (0,1)(Boolean=w860) -> (0, 1=w867:i16)
        n435 = Add(x=w871, y=w869) -> (x+y=w875:u32)
        n436 = To Unsigned Byte Integer(number=w867) -> (unsigned 8bit integer=w864:u8)
        n437 = feedback #39(u8 0) -> (w865:u8)
        n438 = Add(x=w864, y=w865) -> (x+y=w863:u8)
        "MCL Late Counter" <- w863
        n439 = feedback-in #39(w863) -> ()
        "Piezo Y out" <- w858
        "Piezo X out" <- w857
      }
    }
  }
  n440 = while "Trap RF control, main calculations (raster scanning, intensity and position feedback, phase control etc) with primary timing trigger" {
    shift-right: [w900] -> _
    shift-left: w4 -> [w899]
    shift-right: [w898] -> _
    shift-left: FALSE ("Swap F1 and F2") -> [w897]
    shift-right: [w893] -> _
    shift-left: u16 0 ("BD 1 Amplitude 3") -> [w891]
    shift-right: [w890] -> _
    shift-left: u64 0 -> [w889]
    shift-right: [w888] -> _
    shift-left: u64 0 -> [w886]
    shift-right: [w887] -> _
    shift-left: u64 0 -> [w884]
    stop <- FALSE stop-if-true
    n441 = flat-sequence {
      tunnel: w897 -> [w906]
      tunnel: w899 -> [w904]
      tunnel: [w906] -> w896
      tunnel: [w905] -> w895
      tunnel: [w904] -> w894
      tunnel: [w903] -> w892
      tunnel: w891 -> [w903]
      tunnel: [w902] -> w885
      tunnel: w884 -> [w902]
      tunnel: [w919] -> w900
      tunnel: [w918] -> w898
      tunnel: w896 -> [w917]
      tunnel: w895 -> [w916]
      tunnel: w894 -> [w915]
      tunnel: [w914] -> w893
      tunnel: w892 -> [w913]
      tunnel: [w912] -> w890
      tunnel: w889 -> [w911]
      tunnel: [w910] -> w888
      tunnel: [w909] -> w887
      tunnel: w886 -> [w908]
      tunnel: w885 -> [w907]
      frame #0 {
        n442 = call "Loop Timer"("Count(Ticks)"=w904) -> ("Tick Count(Ticks)"=w905:u16)
      }
      frame #1 {
        n443 = flat-sequence {
          tunnel: w917 -> [w925]
          tunnel: w913 -> [w920]
          tunnel: [w969] -> w919
          tunnel: [w981] -> w918
          tunnel: w916 -> [w975]
          tunnel: w915 -> [w972]
          tunnel: [w938] -> w914
          tunnel: [w931] -> w912
          tunnel: w911 -> [w930]
          tunnel: [w929] -> w910
          tunnel: [w928] -> w909
          tunnel: w908 -> [w927]
          tunnel: w907 -> [w926]
          frame #0 {
            w921 = -1 ("Timeout")
            # "Operation when you need a long delay for either X or Y to synchonize AOD light out phase (> ~100 ticks)\nor want shorter trap ON timing. Puts some of the delay timing in parallel with the later computations."
            # "Trigger the external loop by sending the boolean FSK value through a FIFO.\nTiming is precise."
            n444 = Boolean To (0,1)(Boolean=w925) -> (0, 1=w924:i16)
            n445 = To Unsigned Word Integer(number=w924) -> (unsigned 16bit integer=w923:u16)
            n446 = xnode ("FIFO Method Node")("Element"=w923, "Timeout"=w921) -> ("FIFO Out"=w922:refnum<k21>)  [unwired: 1 in, 1 out]
            n447 = xnode ("FIFO Method Node")("Element"=w920, "Timeout"=w921, "FIFO In"=w922) -> ()  [unwired: 2 out]
          }
          frame #1 {
            # "Just counts, wraps around, 8 bit"
            # "Which trap cycle"
            # "Just flips back and forth."
            # "If interlacing is off, this is which cycle to use."
            # "Keep track of trap cycles (trap 1, 2, 3...)"
            # "This is the prior cycle's on time"
            # "increment timing\nindex, reset to 0 if \nend of matrix"
            # "Reset to begginning (1) when number of cycles reached."
            # "timing index"
            # "build byte stacks for writing data\n(must correspond to addresses array constant)"
            # "Timing housekeeping"
            # "Adjust phase if late\n(maintains constant phase relationship between cycles)"
            n448 = feedback #40(u8 0 ("t")) -> (w978:u8)
            n449 = Increment(x=w978) -> (x+1=w1005:u8)
            n450 = Increment(x="Number Interlace Cycles") -> (x+1=w1000:u8)
            n451 = Equal?(x=w1005, y=w1000) -> (x = y?=w1007:bool)
            n452 = Select(t=u8 1, s=w1007, f=w1005) -> (s? t:f=w977:u8)
            n453 = feedback-in #40(w977) -> ()
            n454 = Increment(x=w977) -> (x+1=w1002:u8)
            n455 = Equal?(x=w1002, y=w1000) -> (x = y?=w1003:bool)
            n456 = Select "This cycle"(t=u8 1, s=w1003, f=w1002) -> (s? t:f=w999:u8)
            n457 = Select(t=w999, s="Interlace ON/OFF", f="Interlace Off Parameters") -> (s? t:f=w945:u8)
            n458 = feedback-in #41(w975) -> ()
            n459 = feedback #41(w975) -> (w974:u16)
            n460 = Select(t=w977, s="Interlace ON/OFF", f="Interlace Off Parameters") -> (s? t:f=w998:u8)
            n461 = Subtract(x=w975, y=w974) -> (x-y=w973:u16)
            n462 = Subtract "The error"(x=w973, y=w972) -> (x-y=w956:u16)
            n463 = case shown="1, Default" w998 {
              tunnel: ["DIO count 1 (ticks)" "DIO count 2 (ticks)" "DIO count 3 (ticks)"] -> w971
              frame 1, Default {
              }
              frame 2 {
              }
              frame 3 {
              }
            }
            n464 = Number To Boolean Array(number=w956) -> (Boolean array=w957:bool[])
            n465 = Or Array Elements(Boolean array=w957) -> (logical OR=w955:bool)
            n466 = Boolean To (0,1)(Boolean=w955) -> (0, 1=w962:i16)
            n467 = To Unsigned Byte Integer(number=w962) -> (unsigned 8bit integer=w959:u8)
            n468 = feedback #42(u8 0) -> (w960:u8)
            n469 = Add(x=w959, y=w960) -> (x+y=w958:u8)
            "DIO Late Counter" <- w958
            n470 = feedback-in #42(w958) -> ()
            n471 = Subtract(x=w971, y=w956) -> (x-y=w970:u16)
            n472 = local read "green FB running"() -> (w951:bool)
            n473 = And(x=w951, y="RF synth bd controls green") -> (x .and. y?=w950:bool)
            n474 = case shown="2" w945 {
              tunnel: [w1115 w1324 "BD 1 Frequency 3"] -> w995
              tunnel: [w1112 w1331 "BD 1 Amplitude 3"] -> w938
              tunnel: "FB Gains" -> [w1128 w1334 _]
              tunnel: "FB output range" -> [w1129 w1333 _]
              tunnel: w950 -> [_ _ w1354]
              tunnel: [w1115 w1332 w1353] -> w931
              tunnel: w930 -> [w1114 w1332 w1353]
              tunnel: [w1107 u64 0 u64 0] -> w929
              tunnel: [w1108 u64 0 u64 0] -> w928
              tunnel: w927 -> [_ w1328 _]
              tunnel: w926 -> [_ w1327 _]
              frame 1, Default {
                w1143 = fxp<+/-,24,9> 0.0 ("AI1 X Set 2")
                w1137 = u16 0
                # "Changed by RG:\nenables symmetric motion of \ntraps during raster scanning \nand force feedback."
                # "Changed by Ronen - correction \nby PID is now implemented not on \nthe Base BD1 frequency but on the last\nfrequency sent."
                # "Added by Ronen -\nUpper and Lower \nLimits for the FB \ngenerated frequency\nto avoid losing bead \nwhen tether breaks"
                # "Explanation of raster scanning:\n1. Cycles: increment counter by 1 every time interlace cycle returns to trap 1. As long as \n  Cycle per Step is larger than counter, keep incrementing counter and do not change step counter.\n  Once counter is equal to Cycles per step, zero counter and increment step counter.\n2. Steps: Increments up every time cycles counter equals cycles per step. Performs the following:\n- To determine DIRECTION of frequency change:  If ScanstepX2 is EQUAL to step counter (full for-back scan finished)\n   frequency increment is set to zero, AND step counter is set to zero. \n   Otherwise: if no change to step counter (because cycleperstep>cycle counter), then no change to frequency\n   increment. \n   If step counter has changed (cycleperstep=cycle counter), then need to figure out direction of frequency change:\n   if step counter is EQUAL to Scansteps: No change to frequency increment\n   Otherwise: If scan steps > step counter - 1 (forward scan NOT completed): increment frequency by 1\n                       If scan steps equal or smaller than step counter -1 (forward scan completed): increment frequency by -1\n\n3. Scans: Increment scan counter every time step counter equals 2Xscan steps (full for-back scan completed)\n    if number of scans > scan counter: Send TRUE to scanning, continue scan\n    if number of scans = scan counter: Send FALSE to Scanning, Scan finished.\n\n  The wire with the asterik can be used as the index for getting the mirror positions in the offset scan."
                # "This signal integration happens no matter what\nso that correct setpoints can be chosen before \nturning on the FB."
                # "Trap 1"
                n475 = local read "AI1 X Set 2"() -> (w1126:fxp<+/-,16,1>)
                n476 = local read "AI1 X Set 1"() -> (w1140:fxp<+/-,16,1>)
                n477 = local read "Scanning"() -> (w1156:bool)
                n478 = Multiply(x=w1126, y="B factor") -> (x*y=w1124:fxp<+/-,48,17>)
                n479 = Or(x=w1156, y="Start scan") -> (x .or. y?=w1153:bool)
                n480 = case shown="True" "Diff FB Measurement?" {
                  tunnel: w1124 -> [w1181 w1190]
                  tunnel: w1140 -> [w1180 w1191]
                  tunnel: [w1178 w1182] -> w1141
                  frame False {
                    n481 = Select(t=w1180, s="Trap Pos FB Monitor T1 or T2", f=w1181) -> (s? t:f=w1178:fxp<+/-,48,17>)
                  }
                  frame True {
                    n482 = Subtract(x=w1191, y=w1190) -> (x-y=w1183:fxp<+/-,48,17>)
                    n483 = Not(x="Negate Diff?") -> (.not. x?=w1189:bool)
                    n484 = Boolean To (0,1)(Boolean="Negate Diff?") -> (0, 1=w1187:i16)
                    n485 = Boolean To (0,1)(Boolean=w1189) -> (0, 1=w1188:i16)
                    n486 = Negate(x=w1187) -> (-x=w1186:i16)
                    n487 = Add(x=w1186, y=w1188) -> (x+y=w1184:i16)
                    n488 = Multiply(x=w1184, y=w1183) -> (x*y=w1182:fxp<+/-,63,32>)
                  }
                }
                n489 = Not(x="Abort scan") -> (.not. x?=w1151:bool)
                n490 = And(x=w1151, y=w1153) -> (x .and. y?=w1150:bool)
                n491 = case "For raster scanning" shown="False" w1150 {
                  tunnel: [i64 0 w1314] -> w1110
                  tunnel: "Start scan" -> [_ w1299]
                  tunnel: [u64 1 w1276] -> w1127
                  frame False {
                    n492 = local write "Scanning"(FALSE ("scanning")) -> ()
                  }
                  frame True {
                    w1283 = i64 0
                    w1282 = u64 0
                    # "scan incr."
                    # "freq. incr. mult."
                    # "count steps"
                    # "count number of cycles"
                    n493 = feedback #43(w1282) -> (w1311:u64)
                    n494 = Select(t=w1282, s=w1299, f=w1311) -> (s? t:f=w1313:u64)
                    n495 = Increment(x=w1313) -> (x+1=w1310:u64)
                    n496 = Greater?(x="Cycles per step", y=w1310) -> (0:w1292:bool)
                    n497 = Select(t=w1310, s=w1292, f=w1282) -> (s? t:f=w1309:u64)
                    n498 = feedback-in #43(w1309) -> ()
                    n499 = feedback #44(w1282) -> (w1308:u64)
                    n500 = Select(t=w1282, s=w1299, f=w1308) -> (s? t:f=w1303:u64)
                    n501 = Increment(x=w1303) -> (x+1=w1307:u64)
                    n502 = Add(x="Scan steps", y="Scan steps") -> (x+y=w1306:u64)
                    n503 = Select(t=w1303, s=w1292, f=w1307) -> (s? t:f=w1287:u64)
                    n504 = Greater?(x=w1306, y=w1287) -> (0:w1286:bool)
                    n505 = Select(t=w1287, s=w1286, f=w1282) -> (s? t:f=w1304:u64)
                    n506 = feedback-in #44(w1304) -> ()
                    n507 = Equal?(x="Scan steps", y=w1287) -> (x = y?=w1291:bool)
                    n508 = Greater?(x="Scan steps", y=w1303) -> (0:w1302:bool)
                    n509 = feedback #45(w1283) -> (w1305:i64)
                    n510 = Select(t=w1283, s=w1299, f=w1305) -> (s? t:f=w1289:i64)
                    n511 = Increment(x=w1289) -> (x+1=w1301:i64)
                    n512 = Decrement(x=w1289) -> (x-1=w1300:i64)
                    n513 = Select(t=w1301, s=w1302, f=w1300) -> (s? t:f=w1290:i64)
                    n514 = Select(t=w1289, s=w1291, f=w1290) -> (s? t:f=w1288:i64)
                    n515 = Select(t=w1289, s=w1292, f=w1288) -> (s? t:f=w1284:i64)
                    n516 = Select(t=w1284, s=w1286, f=w1283) -> (s? t:f=w1285:i64)
                    n517 = feedback-in #45(w1285) -> ()
                    n518 = feedback #46(w1282) -> (w1298:u64)
                    n519 = Select(t=w1282, s=w1299, f=w1298) -> (s? t:f=w1294:u64)
                    n520 = Increment(x=w1294) -> (x+1=w1295:u64)
                    n521 = Select(t=w1294, s=w1286, f=w1295) -> (s? t:f=w1293:u64)
                    n522 = Greater?(x="Number of scans", y=w1293) -> (0:w1279:bool)
                    n523 = Multiply(x="Scan freq.  increment", y=w1289) -> (x*y=w1314:i64)
                    n524 = Select(t=TRUE, s="Cont. Scan", f=w1279) -> (s? t:f=w1278:bool)
                    "Scanning" <- w1278
                    n525 = Select(t=w1293, s=w1278, f=w1282) -> (s? t:f=w1296:u64)
                    n526 = feedback-in #46(w1296) -> ()
                    n527 = Increment(x=w1293) -> (x+1=w1276:u64)
                  }
                }
                "Scan I" <- w1127
                n528 = feedback #47(w1137) -> (w1136:u16)
                n529 = Increment(x=w1136) -> (x+1=w1138:u16)
                n530 = Greater Or Equal?(x=w1138, y="Trap Pos FB Int Count") -> (x >= y?=w1113:bool)
                n531 = Select(t=w1137, s=w1113, f=w1138) -> (s? t:f=w1139:u16)
                n532 = feedback-in #47(w1139) -> ()
                n533 = feedback #48(w1143) -> (w1142:fxp<+/-,24,9>)
                n534 = Add(x=w1141, y=w1142) -> (x+y=w1135:fxp<+/-,24,9>)
                n535 = case "Trap 1 X intensity feedback" shown="True" "FB On/Off Set 1" {
                  tunnel: "BD 1 Amplitude 1" -> [w1316 _]
                  tunnel: [w1316 w1320] -> w1112
                  tunnel: w1129 -> [_ w1317]
                  tunnel: w1128 -> [_ w1318]
                  frame False {
                  }
                  frame True {
                    n536 = local read "AI2 Y Sum Set 1"() -> (w1321:i16)
                    n537 = call "Slower PID.vi"("process variable"=w1321, "reset?"="FB Reset Set 1", "setpoint"="FB Setpoint Set 1", "PID gains (x 2^8)"=w1318, "output range"=w1317) -> ("output"=w1322:i16)  [unwired: 10 out]
                    n538 = To Unsigned Word Integer(number=w1322) -> (unsigned 16bit integer=w1320:u16)
                  }
                }
                "BD1 amplitude 1 out" <- w1112
                n539 = Select(t=w1143, s=w1113, f=w1135) -> (s? t:f=w1146:fxp<+/-,24,9>)
                n540 = feedback-in #48(w1146) -> ()
                n541 = Divide(x=w1135, y="Trap Pos FB Int Count") -> (x/y=w1130:fxp<+/-,16,1>)
                n542 = feedback #49(fxp<+/-,24,9> 0.0 ("AI1 X Set 2")) -> (w1147:fxp<+/-,24,9>)
                n543 = Select(t=w1135, s=w1113, f=w1147) -> (s? t:f=w1148:fxp<+/-,24,9>)
                "Trap Pos FB Int Signal" <- w1148
                n544 = feedback-in #49(w1148) -> ()
                n545 = feedback #50(fxp<+/-,16,1> 0.0 ("Trap Pos FB Int-Norm Signal")) -> (w1132:fxp<+/-,16,1>)
                n546 = Select(t=w1130, s=w1113, f=w1132) -> (s? t:f=w1131:fxp<+/-,16,1>)
                "Trap Pos FB Int-Norm Signal" <- w1131
                n547 = feedback-in #50(w1131) -> ()
                n548 = case "For position feedback" shown="True" "Force feedback" {
                  tunnel: [i64 0 w1197] -> w1109
                  tunnel: w1130 -> [_ w1194]
                  tunnel: w1113 -> [_ w1193]
                  frame False {
                  }
                  frame True {
                    n549 = feedback #51(i64 0) -> (w1196:i64)
                    n550 = case shown="True" w1193 {
                      tunnel: [w1198 w1202] -> w1197
                      tunnel: w1196 -> [w1198 _]
                      tunnel: w1194 -> [_ w1201]
                      frame False {
                      }
                      frame True {
                        n551 = xnode ("PID")("process variable"=w1201, "reset?"="Trap Pos. FB Reset", "setpoint"="Trap Pos. FB SP", "PID gains"="Trap Pos. FB Gains", "output range"="Trap pos. FB Range") -> ("output"=w1211:fxp<+/-,16,1>)
                        n552 = Negate(x=w1211) -> (-x=w1210:fxp<+/-,17,2>)
                        n553 = Select(t=w1210, s="Trap Pos FB Negate Action", f=w1211) -> (s? t:f=w1207:fxp<+/-,17,2>)
                        n554 = Scale By Power Of 2(n=u32 15, x=u32 1) -> (x*2^n=w1204:u32)
                        n555 = Multiply(x=w1207, y=w1204) -> (x*y=w1203:fxp<+/-,17,17>)
                        n556 = To Quad Integer(1:w1203) -> (0:w1215:i64)
                        "Trap Pos FB Action" <- w1215
                        n557 = Multiply(x=w1215, y="Trap Pos. FB Mult Factor") -> (x*y=w1213:i64)
                        n558 = Add(x=w1213, y="Trap Pos. FB Offset Factor") -> (x+y=w1202:i64)
                        n559 = disable-structure shown="Disabled" {
                          disable-tunnel: w1202 -> [w1222 _]
                          frame Disabled {
                            w1226 = u32 0
                            n560 = feedback #52() -> (w1223:i64)  [unwired: 1 in]
                            n561 = Add(x=w1222, y=w1223) -> (x+y=w1220:i64)
                            n562 = feedback #53(w1226) -> (w1228:u32)
                            n563 = Increment(x=w1228) -> (x+1=w1217:u32)
                            n564 = Greater Or Equal?(x=w1217, y="FB Trig Integrate") -> (x >= y?=w1218:bool)
                            n565 = Select(t=i64 0, s=w1218, f=w1220) -> (s? t:f=w1224:i64)
                            n566 = feedback-in #52(w1224) -> ()
                            n567 = Select(t=w1226, s=w1218, f=w1217) -> (s? t:f=w1227:u32)
                            n568 = feedback-in #53(w1227) -> ()
                            n569 = And(x=w1218, y="FPGA Trap Trig") -> (x .and. y?=w1225:bool)
                            n570 = case "Trap FB trigger excitation laser ON" shown="True" w1225 {
                              tunnel: w1220 -> [_ w1232]
                              tunnel: w1217 -> [_ w1230]
                              frame False {
                              }
                              frame True {
                                n571 = Not(x="TTrig Negate Pos") -> (.not. x?=w1239:bool)
                                n572 = Boolean To (0,1)(Boolean="TTrig Negate Pos") -> (0, 1=w1237:i16)
                                n573 = Boolean To (0,1)(Boolean=w1239) -> (0, 1=w1238:i16)
                                n574 = Negate(x=w1237) -> (-x=w1236:i16)
                                n575 = Add(x=w1236, y=w1238) -> (x+y=w1235:i16)
                                n576 = Multiply(x=w1235, y=w1232) -> (x*y=w1234:i64)
                                "TTrig Sig" <- w1234
                                n577 = Multiply(x="FPGA TTrig Thresh", y=w1230) -> (x*y=w1231:i64)
                                "TTrig Fin Thresh" <- w1231
                                n578 = Greater Or Equal?(x=w1234, y=w1231) -> (x >= y?=w1233:bool)
                                n579 = case shown="True" w1233 {
                                frame False {
                                }
                                frame True {
                                w1242 = TRUE ("Green FB On/Off")
                                w1244 = u8 2 ("Operating Mode")
                                n580 = local write "Operating Mode 2"(w1244) -> ()
                                n581 = local write "Operating Mode"(w1244) -> ()
                                n582 = local write "Green FB On/Off"(w1242) -> ()
                                n583 = local write "FPGA Trap Trig"(FALSE ("FPGA Trap Trig")) -> ()
                                "TTrig?" <- w1242
                                }
                                }
                              }
                            }
                          }
                          frame Enabled {
                          }
                        }
                      }
                    }
                    n584 = feedback-in #51(w1197) -> ()
                  }
                }
                n585 = case shown="True" "Symmetric force feedback\nand raster scan" {
                  tunnel: [w1160 w1163] -> w1107
                  tunnel: w1110 -> [w1160 w1164]
                  tunnel: [w1159 w1161] -> w1108
                  tunnel: w1109 -> [w1159 w1162]
                  frame False {
                  }
                  frame True {
                    n586 = Scale By Power Of 2(n=i16 -1, x=w1164) -> (x*2^n=w1163:i64)
                    n587 = Scale By Power Of 2(n=i16 -1, x=w1162) -> (x*2^n=w1161:i64)
                  }
                }
                n588 = And(x="Force feedback", y="Dynamic Force FB (Ronen)") -> (x .and. y?=w1121:bool)
                n589 = case shown="False" w1121 {
                  tunnel: w1108 -> [w1169 w1173]
                  tunnel: [w1168 w1172] -> w1120
                  tunnel: w1114 -> [_ w1171]
                  tunnel: w1113 -> [_ w1170]
                  frame False {
                    # "(BD1 Frequency 1)"
                    n590 = Add(x="BD 1 Frequency 1", y=w1169) -> (x+y=w1168:u64)
                  }
                  frame True {
                    n591 = case shown="True" w1170 {
                      tunnel: w1173 -> [_ w1177]
                      tunnel: [w1174 w1176] -> w1172
                      tunnel: w1171 -> [w1174 w1175]
                      frame False {
                      }
                      frame True {
                        n592 = Add(x=w1175, y=w1177) -> (x+y=w1176:u64)
                      }
                    }
                  }
                }
                n593 = Select(t=w1107, s="Scan BD", f=u64 0) -> (s? t:f=w1119:u64)
                n594 = Add(x=w1120, y=w1119) -> (x+y=w1118:u64)
                n595 = In Range and Coerce(upper limit="FB Max Frequency", x=w1118, lower limit="FB Min frequency") -> (coerced(x)=w1115:u64)  [unwired: 1 out]
                "BD1 Frequency Out 1" <- w1115
              }
              frame 2 {
                # "Trap 2"
                n596 = local read "Symmetric force feedback\nand raster scan"() -> (w1330:bool)
                n597 = case shown="True" w1330 {
                  tunnel: "BD 1 Frequency 2" -> [w1337 w1342]
                  tunnel: [w1337 w1338] -> w1324
                  tunnel: w1328 -> [_ w1341]
                  tunnel: w1327 -> [_ w1339]
                  frame False {
                  }
                  frame True {
                    n598 = Subtract(x=w1342, y=w1341) -> (x-y=w1340:u64)
                    n599 = Subtract(x=w1340, y=w1339) -> (x-y=w1338:u64)
                  }
                }
                "BD1 Frequency Out 2" <- w1324
                n600 = case "Trap 2 X intensity feedback" shown="True" "FB On/Off Set 2" {
                  tunnel: [w1343 w1346] -> w1331
                  tunnel: "BD 1 Amplitude 2" -> [w1343 _]
                  tunnel: w1334 -> [_ w1345]
                  tunnel: w1333 -> [_ w1344]
                  frame False {
                  }
                  frame True {
                    n601 = local read "AI2 Y Sum Set 2"() -> (w1349:i16)
                    n602 = call "Slower PID.vi"("process variable"=w1349, "reset?"="FB Reset Set 2", "setpoint"="FB Setpoint Set 2", "PID gains (x 2^8)"=w1345, "output range"=w1344) -> ("output"=w1347:i16)  [unwired: 10 out]
                    n603 = To Unsigned Word Integer(number=w1347) -> (unsigned 16bit integer=w1346:u16)
                  }
                }
                "BD1 amplitude 2 out" <- w1331
              }
              frame 3 {
                # "Fluorescence period"
                n604 = disable-structure shown="Disabled" {
                  disable-tunnel: [w1362 _] -> _
                  disable-tunnel: w1354 -> [w1361 _]
                  frame Disabled {
                    # "Remember if FB was previously on/off"
                    n605 = feedback #54(FALSE) -> (w1357:bool)
                    n606 = case shown="True" w1361 {
                      tunnel: [w1364 w1380] -> w1362
                      tunnel: [w1364 _] -> w1360
                      tunnel: [FALSE TRUE] -> w1358
                      tunnel: w1357 -> [_ w1365]
                      frame False {
                      }
                      frame True {
                        # "Makes it so first time FB run when turned on, the PID sees the detector intensity from the last time FB was running, rather than something near zero. Especially assuming the setpoint is not changing, this will make the FB more stable when resuming, and not overshoot the turnon intensity."
                        # "FB output range: 0 should be low, full scale is 12 bits.\nBut be careful not to go over, then higher bits just get ignored by RF board, so output will actually jump down and be unstable. Keep it under 4000 to be safe."
                        n607 = local read "Green FB Sum"() -> (w1368:i16)
                        n608 = feedback-in #55(w1368) -> ()
                        n609 = feedback #55(i16 0 ("Green FB Sum")) -> (w1367:i16)
                        n610 = Select(t=w1368, s=w1365, f=w1367) -> (s? t:f=w1366:i16)
                        n611 = Bundle("P3 2"="P3 2", "I3 2"="I3 2", "D3 2"="D3 2") -> (w1379:cluster{"P3 2":i16, "I3 2":i16, "D3 2":i16})  [unwired: 1 in]
                        n612 = Bundle("RF synth green feedback max"="RF synth green feedback max", i16 0) -> (w1371:cluster{"RF synth green feedback max":i16, i16})  [unwired: 1 in]
                        n613 = call "Slower PID.vi"("process variable"=w1366, "reset?"="Green FB Reset 2", "setpoint"="Green FB Setpoint 2", "PID gains (x 2^8)"=w1379, "output range"=w1371) -> ("output"=w1381:i16)  [unwired: 10 out]
                        n614 = To Unsigned Word Integer(number=w1381) -> (unsigned 16bit integer=w1380:u16)
                      }
                    }
                    n615 = feedback-in #54(w1358) -> ()
                  }
                  frame Enabled {
                  }
                }
              }
            }
            n616 = Split Number(x=w995) -> (hi(x)=w994:u32, lo(x)=w993:u32)
            n617 = Boolean To (0,1)(Boolean="+ phase (DIO)") -> (0, 1=w967:i16)
            n618 = Split Number(x=w994) -> (lo(x)=w992:u16)  [unwired: 1 out]
            n619 = Split Number(x=w993) -> (hi(x)=w991:u16, lo(x)=w990:u16)
            n620 = Split Number(x=w992) -> (hi(x)=w989:u8, lo(x)=w988:u8)
            n621 = Split Number(x=w991) -> (hi(x)=w987:u8, lo(x)=w986:u8)
            n622 = Split Number(x=w990) -> (hi(x)=w985:u8, lo(x)=w984:u8)
            n623 = Multiply(x=w967, y="Phase count adjustment (DIO)") -> (x*y=w963:i16)
            n624 = feedback #56(TRUE) -> (w953:bool)
            n625 = Not(x=w953) -> (.not. x?=w952:bool)
            n626 = feedback-in #56(w952) -> ()
            n627 = feedback #57(i16 0) -> (w965:i16)
            n628 = Subtract(x=w965, y=w963) -> (x-y=w964:i16)
            "DIO Relative phase" <- w964
            n629 = feedback-in #57(w964) -> ()
            n630 = Add(x=w970, y=w963) -> (x+y=w969:u16)
            n631 = Build Array "BD 1 nu Stack"(w989, w988, w987, w986, w985, w984) -> (w983:u8[])
            n632 = case "Store in RF board F1 or F2" shown="True" w952 {
              tunnel: [w1099 w1102] -> w981
              tunnel: [u8 10 u8 4] -> w982
              tunnel: "Swap F1 and F2" -> [w1100 w1102]
              frame False {
                # "for RF synth controls\ngreen: F1/F2 stay same"
                # "F2 address (hex)"
                n633 = Not(x=w1100) -> (.not. x?=w1099:bool)
              }
              frame True {
                # "low chooses F1"
                # "F1 address (hex)"
              }
            }
            n634 = flat-sequence "Update trap RF synth board settings to be used for the upcoming trap cycle." {
              tunnel: w983 -> [w1062]
              tunnel: [w1062] -> w948
              tunnel: w982 -> [w1063]
              tunnel: w948 -> [w1064]
              tunnel: w939 -> [w1073]
              tunnel: w940 -> [w1072]
              frame #0 {
                # "To possibly delay\nthese writes to very\nend of loop (for x and\ny phase adjust)"
                n635 = call "Wait8"("Count(Ticks)"="Next trap write delay (ticks)") -> ()  [unwired: 1 out]
              }
              frame #1 {
                # "Next trap RF frequency:\n\nWrite next trap cycle frequency to buffer."
                n636 = for {
                  tunnel: w1064 -> [w1069] mode=indexing
                  tunnel: w1063 -> [w1067]
                  i -> [w1068]
                  n637 = To Unsigned Byte Integer(number=w1068) -> (unsigned 8bit integer=w1065:u8)
                  n638 = Add(x=w1067, y=w1065) -> (x+y=w1066:u8)
                  n639 = call "Write to RF Synth Bd1 Only.vi"("Address Byte"=w1066, "BD 1 Byte"=w1069) -> ()  [unwired: 1 in]
                }
              }
              frame #2 {
                # "Send udclk high\n(BD 1 and 2) to make the new frequency active in F1 or F2 word. But it won't actually be the used frequency until FSK switches to it (begining of next cycle)."
                n640 = xnode "FPGA I/O Node"("Connector1/DIO30"=TRUE ("Connector1/DIO15")) -> ()  [unwired: 1 in, 1 out]
              }
              frame #3 {
                n641 = xnode "FPGA I/O Node"("Connector1/DIO30"=FALSE ("Connector1/DIO15")) -> ()  [unwired: 1 in, 1 out]
              }
              frame #4 {
                # "Next trap RF phase offset:\n\nSet the next trap cycle amplitude to the buffer. Won't become active until udclk is set high at proper time at the begining of the next cycle."
                n642 = case shown="True" w1073 {
                  tunnel: w1072 -> [_ w1074]
                  frame False {
                  }
                  frame True {
                    # "phase 1 address start"
                    n643 = for {
                      tunnel: w1074 -> [w1080] mode=indexing
                      tunnel: u8 0 -> [w1078]
                      i -> [w1079]
                      n644 = To Unsigned Byte Integer(number=w1079) -> (unsigned 8bit integer=w1076:u8)
                      n645 = Add(x=w1078, y=w1076) -> (x+y=w1077:u8)
                      n646 = call "Write to RF Synth Bd1 Only.vi"("Address Byte"=w1077, "BD 1 Byte"=w1080) -> ()  [unwired: 1 in]
                    }
                  }
                }
              }
              frame #5 {
                # "Prep to reset RF phase to zero at start of next cycle. Only reset BD 1. Do nothing to BD 2. This puts the settings in the buffer. A udclk high will make both this phase reset and possibly a new phase offset setting active."
                n647 = case shown="True" "RF phase reset before cycles" {
                  frame False {
                  }
                  frame True {
                    w1083 = u8 66  # BD 1 reset
                    n648 = call "write to RF synth bd.vi"("Address Byte"=u8 31, "BD 2 Byte"=u8 2, "BD 1 Byte"=w1083) -> ()
                  }
                }
              }
              frame #6 {
                # "Address"
                # "Data BD 1"
                # "If phase reset wasn't chosen previously, these actions will have no affect. For both BD's, data should be binary 10, and address should be hex 1F (bin 01 1111)"
                # "This sets up the digital communication lines to restart phase accumulation (start RF running agin). It cancels out the possible phase reset. Just need to set WR DIO low then udclk DIOhigh  to make this happen. Doing this here early (and not using the usual board write function) speeds things up.\n\nRestarts RF (BD 1 only, BD2 never stopped in first place)."
                n649 = xnode "FPGA I/O Node"("Connector1/DIO0"=FALSE, "Connector1/DIO1"=FALSE, "Connector1/DIO2"=FALSE, "Connector1/DIO3"=FALSE, "Connector1/DIO4"=FALSE, "Connector1/DIO5"=FALSE, "Connector1/DIO6"=TRUE, "Connector1/DIO7"=FALSE, "Connector1/DIO8"=FALSE, "Connector1/DIO9"=TRUE, "Connector1/DIO10"=TRUE, "Connector1/DIO11"=TRUE, "Connector1/DIO12"=TRUE, "Connector1/DIO13"=TRUE) -> ()  [unwired: 14 in, 14 out]
              }
            }
            n650 = feedback #58(fxp<+,8,8> 0.0) -> (w936:fxp<+,8,8>)
            n651 = Increment(x=w936) -> (x+1=w934:fxp<+,8,8>)
            n652 = feedback-in #58(w934) -> ()
            n653 = case "Trap RF phase offset control methods" shown="3" "Phase offset method" {
              tunnel: [fxp<+,14,14> 0.0 ("Phase BD 1") w1012 w1027 w1056] -> w941
              tunnel: "Phase Trap 1" -> [_ w1013 w1028 _]
              tunnel: w945 -> [_ w1014 w1029 w1057]
              tunnel: [FALSE TRUE TRUE TRUE] -> w939
              tunnel: "Phase Trap 2" -> [_ w1010 w1025 _]
              tunnel: w934 -> [_ _ w1024 _]
              frame 0, Default {
              }
              frame 1 {
                # "Constant increment of phase offset with each trap cycle. This results in a constant phase difference between trap cycles. \nOnly for traps 1 and 2 (set phase offset to zero for set three)."
                n654 = case shown="1, Default" w1014 {
                  tunnel: w1013 -> [_ _ w1020]
                  tunnel: [w1016 fxp<+,14,14> 0.0 w1021] -> w1012
                  tunnel: w1010 -> [w1015 _ _]
                  frame 2 {
                    n655 = feedback #59(fxp<+,14,14> 0.0) -> (w1018:fxp<+,14,14>)
                    n656 = Add(x=w1015, y=w1018) -> (x+y=w1016:fxp<+,14,14>)
                    n657 = feedback-in #59(w1016) -> ()
                  }
                  frame 3 {
                  }
                  frame 1, Default {
                    n658 = feedback #60(fxp<+,14,14> 0.0) -> (w1023:fxp<+,14,14>)
                    n659 = Add(x=w1020, y=w1023) -> (x+y=w1021:fxp<+,14,14>)
                    n660 = feedback-in #60(w1021) -> ()
                  }
                }
              }
              frame 2 {
                # "Changing increment of phase offset with each trap cycle. This results in a constant change in phase difference between trap cycles. \nOnly for traps 1 and 2 (set phase offset to zero for set three)."
                n661 = case shown="2" w1029 {
                  tunnel: w1028 -> [_ _ w1039]
                  tunnel: [w1030 fxp<+,14,14> 0.0 w1037] -> w1027
                  tunnel: w1025 -> [w1032 _ _]
                  tunnel: w1024 -> [w1033 _ w1040]
                  frame 2 {
                    n662 = Multiply(x=w1032, y=w1033) -> (x*y=w1031:fxp<+,16,16>)
                    n663 = feedback #61(fxp<+,14,14> 0.0) -> (w1035:fxp<+,14,14>)
                    n664 = Add(x=w1031, y=w1035) -> (x+y=w1030:fxp<+,14,14>)
                    n665 = feedback-in #61(w1030) -> ()
                  }
                  frame 3 {
                  }
                  frame 1, Default {
                    n666 = Multiply(x=w1039, y=w1040) -> (x*y=w1038:fxp<+,16,16>)
                    n667 = feedback #62(fxp<+,14,14> 0.0) -> (w1042:fxp<+,14,14>)
                    n668 = Add(x=w1038, y=w1042) -> (x+y=w1037:fxp<+,14,14>)
                    n669 = feedback-in #62(w1037) -> ()
                  }
                }
              }
              frame 3 {
                w1049 = u32 1013904223  # LCG constant C (add)
                w1051 = fxp<+,21,21> 1664525.0  # LCG constant A (multiply)
                # "Set a random phase offset. Random number generated using the LCG method. Constants and method taken from NI white noise generator code (method is general though)."
                # "shift to 14 significant bits"
                n670 = feedback #63(u32 4294967295 ("seed")) -> (w1046:u32)
                n671 = Multiply(x=w1046, y=w1051) -> (x*y=w1050:u32)
                n672 = Split Number(x=w1046) -> (hi(x)=w1052:u16)  [unwired: 1 out]
                n673 = To Unsigned Word Integer(number=w1052) -> (unsigned 16bit integer=w1044:u16)
                n674 = Add(x=w1050, y=w1049) -> (x+y=w1048:fxp<+,32,32>)
                n675 = To Unsigned Long Integer(number=w1048) -> (unsigned 32bit integer=w1045:u32)
                n676 = feedback-in #63(w1045) -> ()
                n677 = Scale By Power Of 2(n=i8 -2 ("Uniform scale factor"), x=w1044) -> (x*2^n=w1053:u16)
                n678 = To Fixed-Point(number=w1053) -> (fixed-point=w1043:fxp<+,14,14>)  [unwired: 1 in]
                "Random phase generated" <- w1043
                n679 = case shown="1, Default" w1057 {
                  tunnel: [w1058 fxp<+,14,14> 0.0 w1060] -> w1056
                  tunnel: w1043 -> [w1058 _ w1060]
                  frame 2 {
                  }
                  frame 3 {
                  }
                  frame 1, Default {
                  }
                }
              }
            }
            n680 = To Unsigned Word Integer(number=w941) -> (unsigned 16bit integer=w944:u16)
            n681 = Split Number(x=w944) -> (hi(x)=w942:u8, lo(x)=w943:u8)
            n682 = Build Array ("BD 1 A Stack")(w942, w943) -> (w940:u8[])
          }
        }
      }
    }
  }
  n683 = while "RF synth board interlacing timing loop" {
    tunnel: w4 -> [_]
    stop <- FALSE stop-if-true
    # "This loop is stalled until the RF FIFO get a value. With this method we gain additional delay time (because  we allow the rest of the main RF loop to procede while this loop waits to send the switch signals - a form of parallelism). This helps to simplify the main RF code. \n\nThe code also allow optimal interlacing while also controlling trap RF phase. \n\nNote: a lot of work has gone into optimizing these methods and it is unclear how they can be made any faster or better than this (many failed tries). Right now there is essentially ~4 ticks (~90 ns ns) of imperfection in the switching from trap 1 to trap 2. ~2 ticks of no RF (phase reset) then ~2 ticks of trap 2 with the wrong amplitude (T1 amplitude). The total ticks is 200, so not a big error.\n\nPhase can be precisely set for each trap. Phase reset and switching, has similar delays as fsk frequency switching. And phase reset and phase offset changes are also not simultaneous. So we can't perfectly line everything up.\n\nIf you start from amp zero though (as for trap 1), the on switch is perfect. Likewise the off is perfect for trap 2. \n\nThe green laser switching is also perfect because of its reduced duty cycle and delays in fsk switching between 80 and 0 MHz."
    n684 = xnode ("FIFO Read")("Timeout"=-1) -> ("Element"=w1408:u16, "FIFO Out"=w1405:refnum<k21>)  [unwired: 1 in, 1 out]
    n685 = Equal To 0?(x=w1408) -> (x = 0?=w1406:bool)
    n686 = Not(x=w1406) -> (.not. x?=w1382:bool)
    n687 = flat-sequence "BD 1 and 2 RF phase and amplitude switching" {
      tunnel: w1382 -> [_]
      tunnel: w1400 -> [w1466]
      tunnel: w1399 -> [w1465]
      tunnel: w1398 -> [w1464]
      tunnel: w1397 -> [w1463]
      tunnel: w1396 -> [w1462]
      tunnel: w1395 -> [w1461]
      tunnel: w1394 -> [w1460]
      tunnel: w1393 -> [w1459]
      tunnel: w1392 -> [w1482]
      tunnel: w1391 -> [w1481]
      tunnel: w1390 -> [w1480]
      tunnel: w1389 -> [w1479]
      tunnel: w1388 -> [w1478]
      tunnel: w1387 -> [w1477]
      tunnel: w1386 -> [w1476]
      tunnel: w1385 -> [w1475]
      frame #0 {
        # "Delay to align amp/frequency switching depending on the method used.\n\nCan also give enough time to do the parallel amplitude calculations"
        n688 = call "Wait"("Count(Ticks)"="Amp switch delay") -> ()  [unwired: 1 out]
      }
      frame #1 {
        # "make phase offset and phase reset active with buffer transfer"
        n689 = xnode "FPGA I/O Node"("Connector1/DIO30"=TRUE) -> ()  [unwired: 1 in, 1 out]
      }
      frame #2 {
        w1456 = FALSE ("Connector1/DIO14")
        # "write phase restart to buffer and reset udclk"
        n690 = xnode "FPGA I/O Node"("Connector1/DIO30"=w1456, "Connector1/DIO15"=w1456) -> ()  [unwired: 2 in, 2 out]
      }
      frame #3 {
        w1457 = TRUE ("Connector1/DIO15")
        # "make phase restart active"
        # "reset WR"
        n691 = xnode "FPGA I/O Node"("Connector1/DIO15"=w1457, "Connector1/DIO30"=w1457) -> ()  [unwired: 2 in, 2 out]
      }
      frame #4 {
        # "Address"
        # "set amp byte 1, and reset udclk"
        n692 = xnode "FPGA I/O Node"("Connector1/DIO0"=w1466, "Connector1/DIO1"=w1465, "Connector1/DIO2"=w1464, "Connector1/DIO3"=w1463, "Connector1/DIO4"=w1462, "Connector1/DIO5"=w1461, "Connector1/DIO6"=w1460, "Connector1/DIO7"=w1459, "Connector1/DIO8"=TRUE, "Connector1/DIO9"=FALSE, "Connector1/DIO10"=FALSE, "Connector1/DIO11"=FALSE, "Connector1/DIO12"=FALSE, "Connector1/DIO13"=TRUE, "Connector1/DIO30"=FALSE) -> ()  [unwired: 15 in, 15 out]
      }
      frame #5 {
        # "write amp byte 1 to buffer"
        n693 = xnode "FPGA I/O Node"("Connector1/DIO15"=FALSE ("Connector1/DIO14")) -> ()  [unwired: 1 in, 1 out]
      }
      frame #6 {
        # "reset WR"
        n694 = xnode "FPGA I/O Node"("Connector1/DIO15"=TRUE) -> ()  [unwired: 1 in, 1 out]
      }
      frame #7 {
        # "Address"
        # "set amp byte 2"
        n695 = xnode "FPGA I/O Node"("Connector1/DIO0"=w1482, "Connector1/DIO1"=w1481, "Connector1/DIO2"=w1480, "Connector1/DIO3"=w1479, "Connector1/DIO4"=w1478, "Connector1/DIO5"=w1477, "Connector1/DIO6"=w1476, "Connector1/DIO7"=w1475, "Connector1/DIO8"=TRUE, "Connector1/DIO9"=FALSE, "Connector1/DIO10"=FALSE, "Connector1/DIO11"=FALSE, "Connector1/DIO12"=TRUE, "Connector1/DIO13"=FALSE) -> ()  [unwired: 14 in, 14 out]
      }
      frame #8 {
        # "write amp byte 2"
        n696 = xnode "FPGA I/O Node"("Connector1/DIO15"=FALSE ("Connector1/DIO14")) -> ()  [unwired: 1 in, 1 out]
      }
      frame #9 {
        w1490 = TRUE ("Connector1/DIO14")
        # "transfer amp bytes 1 and 2 and reset WR"
        n697 = xnode "FPGA I/O Node"("Connector1/DIO30"=w1490, "Connector1/DIO15"=w1490) -> ()  [unwired: 2 in, 2 out]
      }
      frame #10 {
        # "reset udclk"
        n698 = xnode "FPGA I/O Node"("Connector1/DIO30"=FALSE ("Connector1/DIO14")) -> ()  [unwired: 1 in, 1 out]
      }
    }
    n699 = flat-sequence "FSK BD 1 (trap X)" {
      tunnel: w1382 -> [w1410]
      tunnel: [w1410] -> w1384
      tunnel: w1384 -> [w1411]
      frame #0 {
        n700 = call "Wait2"("Count(Ticks)"="BD 1 Delay (ticks)") -> ()  [unwired: 1 out]
      }
      frame #1 {
        # "switch frequency"
        n701 = xnode "FPGA I/O Node"("Connector1/DIO36"=w1411) -> ()  [unwired: 1 in, 1 out]
      }
    }
    n702 = xnode ("FIFO Read")("Timeout"=-1, "FIFO In"=w1405) -> ("Element"=w1401:u16)  [unwired: 2 out]
    n703 = node-c288() -> (w1403:T6)  [unwired: 1 in]
    n704 = timed-loop "Convert amplitude words to bits" {
      timing: w1403 -> [_]
      timing-out: [_] -> w1402
      tunnel: w1401 -> [w1440]
      tunnel: [w1428] -> w1400
      tunnel: [w1427] -> w1399
      tunnel: [w1426] -> w1398
      tunnel: [w1425] -> w1397
      tunnel: [w1424] -> w1396
      tunnel: [w1423] -> w1395
      tunnel: [w1422] -> w1394
      tunnel: [w1421] -> w1393
      tunnel: [w1420] -> w1392
      tunnel: [w1419] -> w1391
      tunnel: [w1418] -> w1390
      tunnel: [w1417] -> w1389
      tunnel: [w1416] -> w1388
      tunnel: [w1415] -> w1387
      tunnel: [w1414] -> w1386
      tunnel: [w1413] -> w1385
      stop <- TRUE stop-if-true
      # "Board 1 Data"
      # "Board 1 Data"
      n705 = Split Number(x=w1440) -> (hi(x)=w1439:u8, lo(x)=w1429:u8)
      n706 = Number To Boolean Array(number=w1439) -> (Boolean array=w1449:bool[])
      n707 = Index Array(array=w1449, index=7) -> (element=w1428:bool)
      n708 = Index Array(array=w1449, index=6) -> (element=w1427:bool)
      n709 = Index Array(array=w1449, index=5) -> (element=w1426:bool)
      n710 = Index Array(array=w1449, index=4) -> (element=w1425:bool)
      n711 = Index Array(array=w1449, index=3) -> (element=w1424:bool)
      n712 = Index Array(array=w1449, index=2) -> (element=w1423:bool)
      n713 = Index Array(array=w1449, index=1) -> (element=w1422:bool)
      n714 = Index Array(array=w1449, index=0) -> (element=w1421:bool)
      n715 = Number To Boolean Array(number=w1429) -> (Boolean array=w1438:bool[])
      n716 = Index Array(array=w1438, index=7) -> (element=w1420:bool)
      n717 = Index Array(array=w1438, index=6) -> (element=w1419:bool)
      n718 = Index Array(array=w1438, index=5) -> (element=w1418:bool)
      n719 = Index Array(array=w1438, index=4) -> (element=w1417:bool)
      n720 = Index Array(array=w1438, index=3) -> (element=w1416:bool)
      n721 = Index Array(array=w1438, index=2) -> (element=w1415:bool)
      n722 = Index Array(array=w1438, index=1) -> (element=w1414:bool)
      n723 = Index Array(array=w1438, index=0) -> (element=w1413:bool)
    }
    n724 = node-c288(w1402) -> ()
  }
  n725 = while "Control APD data integration - stream to host" {
    shift-right: [w1495] -> _
    shift-left: w3 -> [w1500]
    stop <- FALSE stop-if-true
    n726 = flat-sequence {
      tunnel: w1500 -> [w1502]
      tunnel: [w1503] -> w1498
      tunnel: [w1502] -> w1496
      tunnel: [w1513] -> w1499
      tunnel: w1498 -> [w1513]
      tunnel: [w1512] -> w1497
      tunnel: w1496 -> [w1512]
      tunnel: [w1511] -> w1494
      tunnel: [w1510] -> w1493
      tunnel: [w1504] -> w1492
      tunnel: [w1561] -> w1495
      tunnel: w1499 -> [w1570]
      tunnel: w1497 -> [w1567]
      tunnel: w1494 -> [w1554]
      tunnel: w1493 -> [w1553]
      tunnel: w1492 -> [w1541]
      frame #0 {
        n727 = call "Loop Timer6"("Count(Ticks)"=w1502) -> ("Tick Count(Ticks)"=w1503:u32)
      }
      frame #1 {
        n728 = flat-sequence {
          tunnel: [w1515] -> w1509
          tunnel: w1509 -> [w1519]
          tunnel: [w1521] -> w1508
          tunnel: [w1520] -> w1507
          tunnel: [w1519] -> w1506
          tunnel: [i16 0] -> w1505
          tunnel: [w1532] -> w1510
          tunnel: [w1533] -> w1511
          tunnel: w1508 -> [w1533]
          tunnel: w1507 -> [w1532]
          tunnel: w1506 -> [w1531]
          tunnel: w1505 -> [w1530]
          tunnel: [w1530] -> w1504
          frame #0 {
            # "use separate variable so each APD won't\nhave to wait to read"
            n729 = feedback #64(FALSE) -> (w1514:bool)
            "APD1 out state" <- w1514
            "APD2 out state" <- w1514
            n730 = disable-structure shown="Disabled" {
              disable-tunnel: w1514 -> [w1517 _]
              frame Disabled {
                "APD3 out state" <- w1517
              }
              frame Enabled {
              }
            }
            n731 = Not(x=w1514) -> (.not. x?=w1515:bool)
            n732 = feedback-in #64(w1515) -> ()
          }
          frame #1 {
            n733 = disable-structure shown="Disabled" {
              disable-tunnel: w1519 -> [w1527 _]
              disable-tunnel: [w1526 _] -> _
              frame Disabled {
                n734 = local read "APD 3 Counts 1"() -> (w1529:u32)
                n735 = local read "APD 3 Counts 0"() -> (w1528:u32)
                n736 = Select(t=w1529, s=w1527, f=w1528) -> (s? t:f=w1526:u32)
              }
              frame Enabled {
              }
            }
            n737 = local read "APD 1 Counts 1"() -> (w1525:u32)
            n738 = local read "APD 1 Counts 0"() -> (w1524:u32)
            n739 = local read "APD 2 Counts 1"() -> (w1523:u32)
            n740 = local read "APD 2 Counts 0"() -> (w1522:u32)
            n741 = Select(t=w1525, s=w1519, f=w1524) -> (s? t:f=w1521:u32)
            n742 = Select(t=w1523, s=w1519, f=w1522) -> (s? t:f=w1520:u32)
          }
          frame #2 {
            n743 = case shown="True" w1531 {
              frame False {
                w1534 = u32 0 ("APD 1 Counts 0")
                n744 = disable-structure shown="Disabled" {
                  disable-tunnel: w1534 -> [w1535 _]
                  frame Disabled {
                    n745 = local write "APD 3 Counts 0"(w1535) -> ()
                  }
                  frame Enabled {
                  }
                }
                n746 = local write "APD 1 Counts 0"(w1534) -> ()
                n747 = local write "APD 2 Counts 0"(w1534) -> ()
              }
              frame True {
                w1536 = u32 0 ("APD 1 Counts 1")
                n748 = disable-structure shown="Disabled" {
                  disable-tunnel: w1536 -> [w1537 _]
                  frame Disabled {
                    n749 = local write "APD 3 Counts 1"(w1537) -> ()
                  }
                  frame Enabled {
                  }
                }
                n750 = local write "APD 1 Counts 1"(w1536) -> ()
                n751 = local write "APD 2 Counts 1"(w1536) -> ()
              }
            }
          }
        }
      }
      frame #2 {
        # "crude initialization: if APD to FIFO is off (usually\nonly before initializing a measurement) count is forced to 0\nand green to true"
        # "count cycles till switching"
        n752 = feedback-in #65(w1570) -> ()
        n753 = feedback #65(w1570) -> (w1569:u32)
        n754 = Subtract(x=w1570, y=w1569) -> (x-y=w1568:u32)
        n755 = Subtract(x=w1568, y=w1567) -> (x-y=w1546:u32)
        n756 = case shown="True" "APD to FIFO" {
          tunnel: w1554 -> [_ w1575]
          tunnel: w1553 -> [_ w1573]
          tunnel: w1541 -> [_ w1571]
          frame False {
          }
          frame True {
            n757 = flat-sequence {
              tunnel: 0 ("Timeout") -> [w1577]
              tunnel: w1575 -> [w1578]
              tunnel: [w1577] -> w1574
              tunnel: w1574 -> [w1579]
              tunnel: w1573 -> [w1580]
              tunnel: [w1579] -> w1572
              tunnel: w1572 -> [w1582]
              tunnel: w1571 -> [w1581]
              frame #0 {
                n758 = xnode ("FIFO Write")("Element"=w1578, "Timeout"=w1577) -> ()  [unwired: 1 in, 2 out]
              }
              frame #1 {
                n759 = xnode ("FIFO Write")("Element"=w1580, "Timeout"=w1579) -> ()  [unwired: 1 in, 2 out]
              }
              frame #2 {
                n760 = xnode ("FIFO Write")("Element"=w1581, "Timeout"=w1582) -> ()  [unwired: 1 in, 2 out]
              }
            }
          }
        }
        n761 = Subtract(x="APD Acq Rate Count", y=w1546) -> (x-y=w1562:u32)
        n762 = Number To Boolean Array(number=w1546) -> (Boolean array=w1547:bool[])
        n763 = Or Array Elements(Boolean array=w1547) -> (logical OR=w1545:bool)
        n764 = Boolean To (0,1)(Boolean=w1545) -> (0, 1=w1552:i16)
        n765 = To Unsigned Byte Integer(number=w1552) -> (unsigned 8bit integer=w1549:u8)
        n766 = feedback #66(u8 0) -> (w1550:u8)
        n767 = Add(x=w1549, y=w1550) -> (x+y=w1548:u8)
        "APD Acq Late Counter" <- w1548
        n768 = feedback-in #66(w1548) -> ()
        n769 = Boolean To (0,1)(Boolean="+ phase (APD Acq)") -> (0, 1=w1558:i16)
        n770 = Multiply(x=w1558, y="Phase Count Adjustment (APD Acq)") -> (x*y=w1555:i16)
        n771 = Add(x=w1562, y=w1555) -> (x+y=w1561:u32)
        n772 = feedback #67(i16 0) -> (w1560:i16)
        n773 = Subtract(x=w1560, y=w1555) -> (x-y=w1557:i16)
        "APD Acq Relative Phase" <- w1557
        n774 = feedback-in #67(w1557) -> ()
        n775 = To Word Integer(number=w1554) -> (16bit integer=w1563:i16)
        n776 = To Word Integer(number=w1541) -> (16bit integer=w1542:i16)
        n777 = To Word Integer(number=w1553) -> (16bit integer=w1564:i16)
        n778 = Multiply(x="APD AO scale factor", y=w1564) -> (x*y=w1543:i16)
        n779 = Multiply(x="APD AO scale factor", y=w1542) -> (x*y=w1539:i16)
        n780 = Multiply(x="APD AO scale factor", y=w1563) -> (x*y=w1544:i16)
        n781 = xnode "FPGA I/O Node"("Connector0/AO5"=w1544, "Connector0/AO7"=w1543, "Connector0/AO6"=w1539) -> ()  [unwired: 3 in, 3 out]
      }
    }
  }
  n782 = disable-structure shown="Disabled" {
    disable-tunnel: w4 -> [w1583 _]
    frame Disabled {
      n783 = while "APD 3 Counter" {
        tunnel: w1583 -> [_]
        stop <- FALSE stop-if-true
        n784 = flat-sequence {
          frame #0 {
            n785 = xnode "FPGA I/O Method Node"("FPGA I/O In"=refnum<k21> "Connector0/DIO12" ("APD 2 DO"), "Timeout"=-1) -> ()  [unwired: 2 out]
          }
          frame #1 {
            n786 = local read "APD3 int gate"() -> (w1587:bool)
            n787 = case shown="True" w1587 {
              frame False {
              }
              frame True {
                n788 = local read "APD3 out state"() -> (w1588:bool)
                n789 = case shown="True" w1588 {
                  frame False {
                    n790 = local read "APD 3 Counts 0"() -> (w1590:u32)
                    n791 = Increment(x=w1590) -> (x+1=→"APD 3 Counts 0":u32)
                  }
                  frame True {
                    n792 = local read "APD 3 Counts 1"() -> (w1592:u32)
                    n793 = Increment(x=w1592) -> (x+1=→"APD 3 Counts 1":u32)
                  }
                }
              }
            }
          }
        }
      }
    }
    frame Enabled {
    }
  }
  n794 = disable-structure shown="Disabled" {
    disable-tunnel: w4 -> [w1594 _]
    disable-tunnel: w5 -> [w1593 _]
    frame Disabled {
      n795 = while "APD 3 Gating" {
        shift-right: [w1598] -> _
        shift-left: w1594 -> [w1603]
        shift-right: [w1597] -> _
        shift-left: w1593 -> [w1595]
        stop <- FALSE stop-if-true
        n796 = flat-sequence {
          tunnel: w1603 -> [w1606]
          tunnel: [w1607] -> w1601
          tunnel: [w1606] -> w1599
          tunnel: [w1605] -> w1596
          tunnel: w1595 -> [w1605]
          tunnel: [w1610] -> w1602
          tunnel: w1601 -> [w1610]
          tunnel: [w1609] -> w1600
          tunnel: w1599 -> [w1609]
          tunnel: w1596 -> [w1608]
          tunnel: [w1631] -> w1598
          tunnel: w1602 -> [w1642]
          tunnel: w1600 -> [w1639]
          tunnel: [w1611] -> w1597
          frame #0 {
            n797 = call "Loop Timer15"("Count(Ticks)"=w1606) -> ("Tick Count(Ticks)"=w1607:u16)
          }
          frame #1 {
            # "Signal maybe then sent through \na transistor before APD"
            n798 = xnode "FPGA I/O Node"("Connector0/DIO2"=w1608) -> ()  [unwired: 1 in, 1 out]
            "APD3 int gate" <- w1608
          }
          frame #2 {
            n799 = local read "APD Gate OFF Count"() -> (w1616:u16)
            n800 = local read "APD Gate ON Count"() -> (w1617:u16)
            n801 = feedback #68(TRUE) -> (w1636:bool)
            n802 = feedback-in #69(w1642) -> ()
            n803 = feedback #69(w1642) -> (w1641:u16)
            n804 = Not(x=w1636) -> (.not. x?=w1634:bool)
            n805 = feedback-in #68(w1634) -> ()
            n806 = Subtract(x=w1642, y=w1641) -> (x-y=w1640:u16)
            n807 = Select(t=w1617, s=w1634, f=w1616) -> (s? t:f=w1638:u16)
            n808 = Subtract(x=w1640, y=w1639) -> (x-y=w1619:u16)
            n809 = Subtract(x=w1638, y=w1619) -> (x-y=w1630:u16)
            n810 = Number To Boolean Array(number=w1619) -> (Boolean array=w1620:bool[])
            n811 = Or Array Elements(Boolean array=w1620) -> (logical OR=w1618:bool)
            n812 = Boolean To (0,1)(Boolean=w1618) -> (0, 1=w1625:i16)
            n813 = Boolean To (0,1)(Boolean="+ phase (APD 3 Gate)") -> (0, 1=w1628:i16)
            n814 = To Unsigned Byte Integer(number=w1625) -> (unsigned 8bit integer=w1622:u8)
            n815 = Multiply(x=w1628, y="Phase count adjustment (APD 3 Gate)") -> (x*y=w1626:i16)
            n816 = feedback #70(u8 0) -> (w1623:u8)
            n817 = Add(x=w1622, y=w1623) -> (x+y=w1621:u8)
            "APD 3 Gate Late Counter" <- w1621
            n818 = feedback-in #70(w1621) -> ()
            n819 = Add(x=w1630, y=w1626) -> (x+y=w1631:u16)
            n820 = feedback #71(i16 0) -> (w1633:i16)
            n821 = Subtract(x=w1633, y=w1626) -> (x-y=w1632:i16)
            "APD 3 Gate Relative Phase" <- w1632
            n822 = feedback-in #71(w1632) -> ()
            n823 = local read "APD Gate Operating Mode"() -> (w1615:u8)
            n824 = case shown="2" w1615 {
              tunnel: [TRUE FALSE w1645] -> w1612
              tunnel: w1636 -> [_ _ w1645]
              frame 0, Default {
              }
              frame 1 {
              }
              frame 2 {
              }
            }
            n825 = local read "Invert APD Gate"() -> (w1614:bool)
            n826 = Not(x=w1612) -> (.not. x?=w1613:bool)
            n827 = Select(t=w1613, s=w1614, f=w1612) -> (s? t:f=w1611:bool)
          }
        }
      }
    }
    frame Enabled {
    }
  }
  n828 = while {
    shift-right: [w1648] -> _
    shift-left: w4 -> [w1654]
    shift-right: [w1649] -> _
    shift-left: _ -> [w1646]
    stop <- FALSE stop-if-true
    n829 = flat-sequence {
      tunnel: w1654 -> [w1657]
      tunnel: [w1658] -> w1652
      tunnel: [w1657] -> w1650
      tunnel: [w1656] -> w1647
      tunnel: w1646 -> [w1656]
      tunnel: [w1661] -> w1653
      tunnel: w1652 -> [w1661]
      tunnel: [w1660] -> w1651
      tunnel: w1650 -> [w1660]
      tunnel: w1647 -> [w1659]
      tunnel: w1653 -> [w1691]
      tunnel: w1651 -> [w1690]
      tunnel: [w1663] -> w1649
      tunnel: [w1662] -> w1648
      frame #0 {
        n830 = call "Loop Timer2"("Count(Ticks)"=w1657) -> ("Tick Count(Ticks)"=w1658:u16)
      }
      frame #1 {
        n831 = xnode "FPGA I/O Node"("Connector0/DIO10"=w1659) -> ()  [unwired: 1 in, 1 out]
      }
      frame #2 {
        n832 = feedback #72(w1691) -> (w1692:u16)
        n833 = feedback-in #72(w1691) -> ()
        n834 = Subtract(x=w1691, y=w1692) -> (x-y=w1693:u16)
        n835 = Subtract(x=w1693, y=w1690) -> (x-y=w1683:u16)
        n836 = Number To Boolean Array(number=w1683) -> (Boolean array=w1688:bool[])
        n837 = Or Array Elements(Boolean array=w1688) -> (logical OR=w1689:bool)
        n838 = Boolean To (0,1)(Boolean="+ phase (EMCCD Gate)") -> (0, 1=w1676:i16)
        n839 = Boolean To (0,1)(Boolean=w1689) -> (0, 1=w1684:i16)
        n840 = To Unsigned Byte Integer(number=w1684) -> (unsigned 8bit integer=w1687:u8)
        n841 = Multiply(x=w1676, y="Phase Count Adjustment EMCCD Gate") -> (x*y=w1678:i16)
        n842 = feedback #73(u8 0) -> (w1686:u8)
        n843 = Add(x=w1687, y=w1686) -> (x+y=w1682:u8)
        "EMCCD Late counter" <- w1682
        n844 = feedback-in #73(w1682) -> ()
        n845 = feedback #74(i16 0) -> (w1677:i16)
        n846 = Subtract(x=w1677, y=w1678) -> (x-y=w1671:i16)
        "EMCCD relative phase" <- w1671
        n847 = feedback-in #74(w1671) -> ()
        n848 = feedback #75(TRUE) -> (w1669:bool)
        n849 = Not(x=w1669) -> (.not. x?=w1667:bool)
        n850 = Select(t="EMCCD Gate ON count", s=w1667, f="EMCCD Gate OFF count") -> (s? t:f=w1679:u16)
        n851 = Subtract(x=w1679, y=w1683) -> (x-y=w1672:u16)
        n852 = Add(x=w1672, y=w1678) -> (x+y=w1662:u16)
        n853 = feedback-in #75(w1667) -> ()
        n854 = case shown="1" "EMCCD Gate Operating Mode" {
          tunnel: w1667 -> [_ _ w1696]
          tunnel: [TRUE FALSE w1696] -> w1665
          frame 0, Default {
          }
          frame 1 {
          }
          frame 2 {
          }
        }
        n855 = Not(x=w1665) -> (.not. x?=w1666:bool)
        n856 = Select(t=w1666, s="Invert EMCCD Gate", f=w1665) -> (s? t:f=w1663:bool)
      }
    }
  }
  n857 = disable-structure shown="Disabled" {
    disable-tunnel: w4 -> [w1699 _]
    disable-tunnel: w15 -> [w1698 _]
    frame Disabled {
      n858 = while "633 nm red  fluorescent laser interlacing (DO to IA 633 nm AOM ME amp)." {
        shift-right: [w1820] -> _
        shift-left: w1699 -> [w1825]
        shift-right: [w1819] -> _
        shift-left: w1698 -> [w1817]
        stop <- FALSE stop-if-true
        n859 = flat-sequence {
          tunnel: w1825 -> [w1828]
          tunnel: [w1829] -> w1823
          tunnel: [w1828] -> w1821
          tunnel: [w1827] -> w1818
          tunnel: w1817 -> [w1827]
          tunnel: [w1832] -> w1824
          tunnel: w1823 -> [w1832]
          tunnel: [w1831] -> w1822
          tunnel: w1821 -> [w1831]
          tunnel: w1818 -> [w1830]
          tunnel: [w1841] -> w1820
          tunnel: w1824 -> [w1861]
          tunnel: w1822 -> [w1858]
          tunnel: [w1850] -> w1819
          frame #0 {
            n860 = call "Loop Timer11"("Count(Ticks)"=w1828) -> ("Tick Count(Ticks)"=w1829:u16)
          }
          frame #1 {
            # "Then to PRL 440 amp"
            n861 = xnode "FPGA I/O Node"("Connector1/DIO32"=w1830) -> ()  [unwired: 1 in, 1 out]
          }
          frame #2 {
            n862 = feedback-in #76(w1861) -> ()
            n863 = feedback #76(w1861) -> (w1860:u16)
            n864 = Subtract(x=w1861, y=w1860) -> (x-y=w1859:u16)
            n865 = Subtract(x=w1859, y=w1858) -> (x-y=w1834:u16)
            n866 = Number To Boolean Array(number=w1834) -> (Boolean array=w1835:bool[])
            n867 = Or Array Elements(Boolean array=w1835) -> (logical OR=w1833:bool)
            n868 = Boolean To (0,1)(Boolean="+ phase (RI)") -> (0, 1=w1846:i16)
            n869 = Multiply(x=w1846, y="Phase count adjustment (RI)") -> (x*y=w1843:i16)
            n870 = Boolean To (0,1)(Boolean=w1833) -> (0, 1=w1840:i16)
            n871 = To Unsigned Byte Integer(number=w1840) -> (unsigned 8bit integer=w1837:u8)
            n872 = feedback #77(i16 0) -> (w1844:i16)
            n873 = feedback #78(u8 0) -> (w1838:u8)
            n874 = Add(x=w1837, y=w1838) -> (x+y=w1836:u8)
            "RI Late Counter" <- w1836
            n875 = feedback-in #78(w1836) -> ()
            n876 = Subtract(x=w1844, y=w1843) -> (x-y=w1842:i16)
            "RI Relative phase" <- w1842
            n877 = feedback-in #77(w1842) -> ()
            n878 = feedback #79(TRUE) -> (w1853:bool)
            n879 = case shown="2" "Red Laser Operating Mode" {
              tunnel: [TRUE FALSE w1867] -> w1850
              tunnel: w1853 -> [_ _ w1864]
              frame 0, Default {
              }
              frame 1 {
              }
              frame 2 {
                n880 = Not(x=w1864) -> (.not. x?=w1866:bool)
                n881 = Select(t=w1866, s="Invert RI", f=w1864) -> (s? t:f=w1867:bool)
              }
            }
            n882 = Not(x=w1853) -> (.not. x?=w1849:bool)
            n883 = Select(t="Red interlace ON count", s=w1849, f="Red interlace OFF count") -> (s? t:f=w1855:u16)
            n884 = Subtract(x=w1855, y=w1834) -> (x-y=w1847:u16)
            n885 = Add(x=w1847, y=w1843) -> (x+y=w1841:u16)
            n886 = feedback-in #79(w1849) -> ()
          }
        }
      }
      n887 = while "473 nm blue  fluorescent laser interlacing (DO to blue laser digital control input)." {
        shift-right: [w1716] -> _
        shift-left: w1699 -> [w1719]
        shift-right: [w1715] -> _
        shift-left: w1698 -> [w1713]
        shift-right: [w1708] -> _
        shift-left: _ -> [w1707]
        shift-right: [w1700] -> _
        shift-left: u16 0 -> [w1703]
        stop <- FALSE stop-if-true
        n888 = flat-sequence {
          tunnel: w1719 -> [w1724]
          tunnel: [w1725] -> w1718
          tunnel: [w1724] -> w1717
          tunnel: [w1723] -> w1714
          tunnel: w1713 -> [w1723]
          tunnel: w1707 -> [w1722]
          tunnel: [w1722] -> w1706
          tunnel: [w1721] -> w1704
          tunnel: w1703 -> [w1721]
          tunnel: [w1730] -> w1712
          tunnel: w1718 -> [w1730]
          tunnel: [w1729] -> w1711
          tunnel: w1717 -> [w1729]
          tunnel: w1714 -> [w1728]
          tunnel: w1706 -> [w1727]
          tunnel: [w1727] -> w1705
          tunnel: w1704 -> [w1726]
          tunnel: [w1726] -> w1702
          tunnel: [w1735] -> w1710
          tunnel: [w1734] -> w1709
          tunnel: w1711 -> [w1734]
          tunnel: w1712 -> [w1735]
          tunnel: w1705 -> [w1733]
          tunnel: w1702 -> [w1732]
          tunnel: [w1731] -> w1701
          tunnel: [w1792] -> w1716
          tunnel: w1710 -> [w1810]
          tunnel: w1709 -> [w1807]
          tunnel: [w1780] -> w1715
          tunnel: [w1778] -> w1708
          tunnel: w1701 -> [w1775]
          tunnel: [w1776] -> w1700
          frame #0 {
            n889 = call "Loop Timer14"("Count(Ticks)"=w1724) -> ("Tick Count(Ticks)"=w1725:u16)
          }
          frame #1 {
            n890 = xnode "FPGA I/O Node"("Connector1/DIO28"=w1728) -> ()  [unwired: 1 in, 1 out]
          }
          frame #2 {
            n891 = case shown="True" w1733 {
              tunnel: w1732 -> [w1736 w1738]
              tunnel: [w1736 w1737] -> w1731
              frame False {
              }
              frame True {
                n892 = flat-sequence {
                  tunnel: [w1744] -> w1741
                  tunnel: [w1743] -> w1740
                  tunnel: [w1742] -> w1739
                  tunnel: w1738 -> [w1742]
                  tunnel: w1741 -> [w1761]
                  tunnel: w1740 -> [w1758]
                  tunnel: w1739 -> [w1760]
                  tunnel: [w1759] -> w1737
                  frame #0 {
                    # "5 ns timing resolution"
                    n893 = node-c288() -> (w1747:T6)  [unwired: 1 in]
                    n894 = timed-loop {
                      timing: w1747 -> [_]
                      timing-out: [_] -> w1746
                      tunnel: "Lifetime timeout APD1" -> [w1753]
                      tunnel: [w1748] -> w1743
                      tunnel: [w1749] -> w1744
                      i -> [w1750]
                      stop <- w1752 stop-if-true
                      n895 = xnode "FPGA I/O Node"() -> ("Connector0/DIO5"=w1751:bool)  [unwired: 1 in, 1 out]
                      n896 = To Unsigned Word Integer(number=w1750) -> (unsigned 16bit integer=w1748:u16)
                      n897 = Equal?(x=w1753, y=w1748) -> (x = y?=w1749:bool)
                      n898 = Or(x=w1751, y=w1749) -> (x .or. y?=w1752:bool)
                    }
                    n899 = node-c288(w1746) -> ()
                  }
                  frame #1 {
                    n900 = Not(x=w1761) -> (.not. x?=w1762:bool)
                    n901 = case shown="True" w1762 {
                      tunnel: w1758 -> [_ w1764]
                      tunnel: w1760 -> [w1763 w1766]
                      tunnel: [w1763 w1765] -> w1759
                      frame False {
                        # "timed out, do nothing"
                      }
                      frame True {
                        # "photon detected,record time"
                        n902 = case shown="True" "Lifetime to FIFO" {
                          tunnel: w1764 -> [_ w1772]
                          tunnel: w1766 -> [w1768 w1770]
                          tunnel: [w1768 w1769] -> w1765
                          frame False {
                            # "don't record time\n(can't if doing force feedback)"
                          }
                          frame True {
                            # "number of events in fifo"
                            n903 = xnode ("FIFO Method Node")("Element"=w1772, "Timeout"=0) -> ()  [unwired: 1 in, 2 out]
                            n904 = Increment(x=w1770) -> (x+1=w1769:u16)
                          }
                        }
                        "lifetime (ticks)" <- w1764
                      }
                    }
                  }
                }
              }
            }
          }
          frame #3 {
            # "Reading fifo is tricky here since\nunknown # of events"
            # "For lifetime measurement:\nInterlacing and pulse falling"
            n905 = feedback-in #80(w1810) -> ()
            n906 = feedback #80(w1810) -> (w1809:u16)
            n907 = Subtract(x=w1810, y=w1809) -> (x-y=w1808:u16)
            n908 = Subtract(x=w1808, y=w1807) -> (x-y=w1785:u16)
            n909 = Number To Boolean Array(number=w1785) -> (Boolean array=w1786:bool[])
            n910 = Or Array Elements(Boolean array=w1786) -> (logical OR=w1784:bool)
            n911 = Boolean To (0,1)(Boolean="+ phase (BI D)") -> (0, 1=w1797:i16)
            n912 = Multiply(x=w1797, y="Phase count adjustment (BI D)") -> (x*y=w1794:i16)
            n913 = Boolean To (0,1)(Boolean=w1784) -> (0, 1=w1791:i16)
            n914 = To Unsigned Byte Integer(number=w1791) -> (unsigned 8bit integer=w1788:u8)
            n915 = feedback #81(i16 0) -> (w1795:i16)
            n916 = feedback #82(u8 0) -> (w1789:u8)
            n917 = Add(x=w1788, y=w1789) -> (x+y=w1787:u8)
            "Blue Late Counter (D)" <- w1787
            n918 = feedback-in #82(w1787) -> ()
            n919 = Subtract(x=w1795, y=w1794) -> (x-y=w1793:i16)
            "BI Relative phase (D)" <- w1793
            n920 = feedback-in #81(w1793) -> ()
            n921 = feedback #83(TRUE) -> (w1802:bool)
            n922 = case shown="2" "Blue Laser Operating Mode (D)" {
              tunnel: [TRUE FALSE w1816] -> w1780
              tunnel: w1802 -> [_ _ w1813]
              frame 0, Default {
              }
              frame 1 {
              }
              frame 2 {
                n923 = Not(x=w1813) -> (.not. x?=w1815:bool)
                n924 = Select(t=w1815, s="Invert BI (D)", f=w1813) -> (s? t:f=w1816:bool)
              }
            }
            n925 = Subtract(x=w1775, y="Lifetime events to read blue") -> (x-y=w1773:u16)
            n926 = Not(x=w1802) -> (.not. x?=w1800:bool)
            n927 = Select(t="Blue interlace ON count (D)", s=w1800, f="Blue interlace OFF count (D)") -> (s? t:f=w1804:u16)
            n928 = Subtract(x=w1804, y=w1785) -> (x-y=w1798:u16)
            n929 = Add(x=w1798, y=w1794) -> (x+y=w1792:u16)
            n930 = feedback-in #83(w1800) -> ()
            n931 = Select(t=w1773, s="Lifetime read blue fifo", f=w1775) -> (s? t:f=w1776:u16)
            "lifetime events in fifo" <- w1776
            n932 = Equal?(x="Blue Laser Operating Mode (D)", y=u8 2) -> (x = y?=w1781:bool)
            n933 = Not(x=w1780) -> (.not. x?=w1779:bool)
            n934 = And(x=w1779, y=w1781) -> (x .and. y?=w1778:bool)
          }
        }
      }
    }
    frame Enabled {
    }
  }
